vi "Actor Core.vi"(8 "error in":errorcluster, 11 "SinglePhotonInterferenceUI in":refnum<class "SinglePhotonInterferenceUI.lvclass">) -> (0 "error out":errorcluster, 3 "Actor out":refnum<class "Actor.lvclass">)   [LabVIEW 2023, in "SinglePhoton Library.lvlib" / "SinglePhotonInterferenceUI.lvlib" / "SinglePhotonInterferenceUI.lvclass"]
doc: "(<B>Filename</B>: Actor Framework.lvlib:Actor.lvclass:Actor Core.vi)\n\nReceives messages to the actor, reacts to them, and initiates any error handling that may shut the actor down.\n\nDescendant classes may override this VI to append parallel tasks for the actor to complete while it handles messages. Overrides use the Call Parent Class Method node."
uses:
  SinglePhotonInterferenceUI.lvclass
  C:/Program Files/National Instruments/LabVIEW 2023/vi.lib/ActorFramework/Actor/Actor.lvclass
  <vilib>/ActorFramework/Actor/Actor.lvclass
  ConcreteClasses/ConcreteInstrumentClasses/Multiharp/Multiharp/Types/MH_InputChannel.ctl
  ConcreteClasses/ConcreteInstrumentClasses/Multiharp/Multiharp/_lib/PQ/MultiHarp/MH_MeasMode.ctl
  <vilib>/ActorFramework/Message Enqueuer/Message Enqueuer.lvclass
  ConcreteClasses/ConcreteInstrumentClasses/Multiharp/Multiharp/Types/MH_UIThread_Data_SPI.ctl
  ConcreteClasses/ConcreteInstrumentClasses/Multiharp/Multiharp/_lib/PQ/MultiHarp/MH_InitInfo.ctl
  ConcreteClasses/ConcreteInstrumentClasses/Multiharp/Multiharp/Types/MH_SetInpChanData.ctl
  ConcreteClasses/ConcreteInstrumentClasses/Multiharp/Multiharp/Types/MH_SetInpChanCmds.ctl
  ConcreteClasses/ConcreteInstrumentClasses/Multiharp/Multiharp/Multiharp/Multiharp.lvclass
  <vilib>/ActorFramework/Actor/Actor.lvclass/Actor.ctl
  <vilib>/ActorFramework/Message Enqueuer/Message Enqueuer.lvclass/Message Enqueuer.ctl
  SinglePhotonInterferenceUI.lvclass/SinglePhotonInterferenceUI.ctl
  ConcreteClasses/ConcreteInstrumentClasses/Multiharp/Multiharp/Multiharp Messages/MH_Init Msg/MH_Init Msg.lvclass/MH_Init Msg.ctl
  ConcreteClasses/ConcreteInstrumentClasses/Multiharp/Multiharp/Multiharp Messages/SetInputChannels Msg/SetInputChannels Msg.lvclass/SetInputChannels Msg.ctl
  SPIController/SPIController Messages/MeasurementFinished Msg/MeasurementFinished Msg.lvclass/MeasurementFinished Msg.ctl
  ConcreteClasses/ConcreteInstrumentClasses/Multiharp/Multiharp/Multiharp Messages/SetSyncDivider Msg/SetSyncDivider Msg.lvclass/SetSyncDivider Msg.ctl
  ConcreteClasses/ConcreteInstrumentClasses/Multiharp/Multiharp/Multiharp Messages/SetSyncOffset Msg/SetSyncOffset Msg.lvclass/SetSyncOffset Msg.ctl
  ConcreteClasses/ConcreteInstrumentClasses/Multiharp/Multiharp/Multiharp Messages/SetSyncTrigger Msg/SetSyncTrigger Msg.lvclass/SetSyncTrigger Msg.ctl
  ConcreteClasses/ConcreteInstrumentClasses/Multiharp/Multiharp/Multiharp Messages/SetSyncDeadTime Msg/SetSyncDeadTime Msg.lvclass/SetSyncDeadTime Msg.ctl
  ConcreteClasses/ConcreteInstrumentClasses/Multiharp/Multiharp/Multiharp Messages/SetHistogramParameter Msg/SetHistogramParameter Msg.lvclass/SetHistogramParameter Msg.ctl
  ConcreteClasses/ConcreteInstrumentClasses/Multiharp/Multiharp/Multiharp Messages/MH_SetHistoOnOff Msg/MH_SetHistoOnOff Msg.lvclass/MH_SetHistoOnOff Msg.ctl
  <vilib>/ActorFramework/Message Enqueuer/Init from Existing Queue.vi
  <vilib>/ActorFramework/Message Enqueuer/Enqueue.vi
  ConcreteClasses/ConcreteInstrumentClasses/Multiharp/Multiharp/Multiharp Messages/MH_Init Msg/MH_Init Msg.lvclass
  C:/Program Files/National Instruments/LabVIEW 2023/vi.lib/ActorFramework/Message/Message.lvclass
  ConcreteClasses/ConcreteInstrumentClasses/Multiharp/Multiharp/Multiharp Messages/SetInputChannels Msg/SetInputChannels Msg.lvclass
  SPIController/SPIController Messages/MeasurementFinished Msg/MeasurementFinished Msg.lvclass
  ConcreteClasses/ConcreteInstrumentClasses/Multiharp/Multiharp/Multiharp Messages/StopMeasurement Msg/StopMeasurement Msg.lvclass
  ConcreteClasses/ConcreteInstrumentClasses/Multiharp/Multiharp/Multiharp Messages/SetSyncDivider Msg/SetSyncDivider Msg.lvclass
  ConcreteClasses/ConcreteInstrumentClasses/Multiharp/Multiharp/Multiharp Messages/SetSyncOffset Msg/SetSyncOffset Msg.lvclass
  ConcreteClasses/ConcreteInstrumentClasses/Multiharp/Multiharp/Multiharp Messages/SetSyncTrigger Msg/SetSyncTrigger Msg.lvclass
  ConcreteClasses/ConcreteInstrumentClasses/Multiharp/Multiharp/Multiharp Messages/SetSyncDeadTime Msg/SetSyncDeadTime Msg.lvclass
  ConcreteClasses/ConcreteInstrumentClasses/Multiharp/Multiharp/Multiharp Messages/SetHistogramParameter Msg/SetHistogramParameter Msg.lvclass
  ConcreteClasses/ConcreteInstrumentClasses/Multiharp/Multiharp/Multiharp Messages/MH_SetHistoOnOff Msg/MH_SetHistoOnOff Msg.lvclass
  <vilib>/ActorFramework/Stop Msg/Stop Msg.lvclass
  <vilib>/Utility/error.llb/Error Cluster From Error Code.vi
  ConcreteClasses/ConcreteInstrumentClasses/Multiharp/Multiharp/_lib/PQ/MultiHarp/mhlib_x86_x64_AnyThread.llb/MH_DllPath_global.vi
  <vilib>/ActorFramework/Message Priority Queue/Priority Enqueue.vi
  <vilib>/ErrorRing/Error Ring.xnode
  typedefs/typedefs.lvlib
panel:
  in  "MH_UIThread_Data":T1={"Init Info"={"Library Version"="", "Serial No."="", "Model"="", "Partnum"="", "Version"="", "features"=0, "nchannels"=0, "Base Resolution"=0.0, "Bin Steps"=0}, "DevIdx"=0, "SyncDivider"=1, "SyncOffset"=0, "SyncLevel"=50, "Channels"=[], "CurrentChannels"=[], "AcqTime"=1, "Binning"=1, "HistoOffset"=1, "HistoLen"=1024, "StopOvl."=FALSE, "OvlLevel"=1024, "SyncEdge"=10, "StartMeas"=FALSE, "HistoLength"=0, "Resolution"=0.0, "Run cont."=FALSE, "Status"="", "SyncRate"=0, "BitShift"=0, "HistoAcqTime"=0.0, "SyncRateStart"=0, "UseDeadTime"=FALSE, "SyncDeadTime"=800, "SetInpChan"=[], "max value"=[], "CoincidenceArray"=[], "Histo On"=FALSE, "Mode"=0, "Scanning"=FALSE, "Last Move"=FALSE, "Coincidence Window"=0.0, "Max Triggers"=0, "Coincidence Delays"=[], "T2 Coincidences Array"=[], "Clear Graph"=FALSE, "File Save Path"=path "", "T2 Coincidence Cluster"={"Coincidences"=[], "Mean"=[], "Sqrt(mean)"=[], "Stdev"=[]}, "Acquisitions"=0, "HR Array"=[], "Ext. Scanning"=FALSE, "AllanVariance"=[]} {"Acquisitions" min=0 max=100000000 step=1; "T2 Coincidence Cluster"."Stdev" format="%0.2f"; "T2 Coincidence Cluster"."Mean" format="%0.2f"; "Mode" items=["HIST"=0, "T2"=2, "T3"=3]; "SyncDeadTime" min=800 max=160000 step=1; "SyncEdge" items=["falling", "rising"]; "SyncDivider" items=["1", "2", "4", "8", "16"]; "SyncOffset" min=0 max=100000 step=1; "SyncLevel" min=0 max=800 step=1; "AcqTime" min=1 max=360000 step=1; "Binning" items=["1", "2", "4", "8", "16", "32", "64", "128", "256", "512", "1024", "2048", "4096", "8192", "16384", "32768", "65536", "131072", "262144", "524288", "1048576", "2097152", "4194304", "8388608", "16777216", "3355443225"]; "HistoOffset" min=0 max=500 step=1; "HistoLen" min=1024 max=65536 step=1024; "Channels"."DeadTime" min=800 max=160000 step=1; "Channels"."Edge" items=["falling", "rising"]; "Channels"."Offset" min=-100000 max=100000 step=10; "Channels"."Level" min=-1200 max=1200 step=1}
  out "Self Enqueuer":refnum<class "Message Enqueuer.lvclass">
  out "Caller Enqueuer":refnum<class "Message Enqueuer.lvclass">
  out "Multiharp Enqueuer":refnum<class "Message Enqueuer.lvclass">
  out "T2 Coincidence Cluster.Coincidences":i32[][](graph)
  out "AllanVariance":dbl[][](graph)
  out "syncrate":i32
  in  "Histograms On":bool
  in  "Acquisitions":u32=1 min=1 max=5000 step=1
  out "T2 Coincidence Cluster":T7 {"Stdev" format="%0.2f"; "Mean" format="%0.2f"}
  in  "FileName":string
  in  "Path":path
  in  "Clear Graph":bool
  in  "Coincidence Delays":dbl[](array[numeric])
  in  "Max Triggers":i32
  in  "Coincidence Window":dbl
  in  "Mode":T6=2 items=["HIST"=0, "T2"=2, "T3"=3]
  in  "HistoLength":i32(ring)=6 caption="Num Bins" items=["1024", "2048", "4096", "8192", "16384", "32768", "65536"]
  out "Status":string="Readout Rate: 8.6 Hz\t\tTotal Counts:\t\tCh. 1: 0 cnts.\t\tCh. 2: 1962112 cnts.\t\tCh. 3: 0 cnts.\t\tCh. 4: 1962112 cnts.\t\tCh. 5: 0 cnts.\t\tCh. 6: 1962112 cnts.\t\tCh. 7: 0 cnts.\t\tCh. 8: 1962112 cnts.\t\tCh. 9: 1962113 cnts.\t\tCh.10: 0 cnts.\t\tCh.11: 1962113 cnts.\t\tCh.12: 0 cnts.\t\tCh.13: 1962113 cnts.\t\tCh.14: 0 cnts.\t\tCh.15: 1962113 cnts.\t\tCh.16: 1962113 cnts.\t\t"
  out "CountRates":i32[](graph)
  out "SyncRate":string="Sync Rate: 4999950 cps\n"
  out "OverFlow":bool caption="Overflow:"
  out "HistoGraph":T8(graph)={0.0, "Resolution"=0.08, "Histograms"=[]}
  in  "AllChannels":T9={"Enable"=TRUE, "Offset"=0, "Level"=20, "Edge"=0, "DeadTime"=1000, "UseDeadTime"=FALSE, "SetEnableAllChan"=TRUE, "SetEdgeAllChan"=TRUE, "SetLevelAllChan"=TRUE, "SetOffsetAllChan"=TRUE, "SetUseDTAllChan"=TRUE, "SetDeadTAllChan"=TRUE} {"DeadTime" min=800 max=160000 step=1; "Edge" items=["falling", "rising"]; "Offset" min=-100000 max=100000 step=10; "Level" min=-1200 max=1200 step=1}
  in  "Scale":enum32{"Item 0", "Item 1"}(radio)
  in  "Run continuously":enum32{"Running Mode", "Item 1"}(radio) caption="Acquisition"
  in  "Start":bool
  in  "OvlLevel":u32=4294967295 caption="Ovl.Level" min=1 step=1
  in  "StopOvl.":bool=TRUE
  in  "AcqTime":i32=1000 caption="Acqu.           ms" min=1 max=3600000 step=1
  in  "HistoOffset":i32 caption="Offset            ns" min=0 max=100000000 step=1
  in  "Binning":i32(ring) caption="Resol.            ps" items=["10", "20", "40", "80", "160", "320", "640", "1280", "2560", "5120", "10240", "20480", "40960", "81920", "163840", "327680", "655360", "1310720", "2621440", "5242880", "10485760", "20971520", "41943040"]
  in  "UseDeadTime":bool caption="Use DT."
  in  "SyncDeadTime":i32=1000 caption="Dead T.   ps" min=800 max=160000 step=1
  in  "SyncLevel":i32=-100 caption="Level      mV" min=-1200 max=1200 step=1
  in  "SyncEdge":i32(ring) caption="Edge" items=["falling", "rising"]
  in  "SyncOffset":i32 caption="Offset      ps" min=-100000 max=100000 step=10
  in  "SyncDivider":i32(ring) caption="Divider" items=["1", "2", "4", "8", "16"]
  in  "Channels":T3[](array[typedef])=[{"Name"="Inp.Chan 1", "Enable"=TRUE, "Edge"=0, "Level"=-100, "Offset"=0, "UseDeadTime"=FALSE, "DeadTime"=1000}, {"Name"="Inp.Chan 2", "Enable"=TRUE, "Edge"=0, "Level"=-100, "Offset"=0, "UseDeadTime"=FALSE, "DeadTime"=1000}, {"Name"="Inp.Chan 3", "Enable"=TRUE, "Edge"=0, "Level"=-100, "Offset"=0, "UseDeadTime"=FALSE, "DeadTime"=1000}, {"Name"="Inp.Chan 4", "Enable"=TRUE, "Edge"=0, "Level"=-100, "Offset"=0, "UseDeadTime"=FALSE, "DeadTime"=1000}, {"Name"="Inp.Chan 5", "Enable"=TRUE, "Edge"=0, "Level"=-100, "Offset"=0, "UseDeadTime"=FALSE, "DeadTime"=1000}, {"Name"="Inp.Chan 6", "Enable"=TRUE, "Edge"=0, "Level"=-100, "Offset"=0, "UseDeadTime"=FALSE, "DeadTime"=1000}, {"Name"="Inp.Chan 7", "Enable"=TRUE, "Edge"=0, "Level"=-100, "Offset"=0, "UseDeadTime"=FALSE, "DeadTime"=1000}, {"Name"="Inp.Chan 8", "Enable"=TRUE, "Edge"=0, "Level"=-100, "Offset"=0, "UseDeadTime"=FALSE, "DeadTime"=1000}, {"Name"="Inp.Chan 9", "Enable"=TRUE, "Edge"=0, "Level"=-100, "Offset"=0, "UseDeadTime"=FALSE, "DeadTime"=1000}, {"Name"="Inp.Chan 10", "Enable"=TRUE, "Edge"=0, "Level"=-100, "Offset"=0, "UseDeadTime"=FALSE, "DeadTime"=1000}, {"Name"="Inp.Chan 11", "Enable"=TRUE, "Edge"=0, "Level"=-100, "Offset"=0, "UseDeadTime"=FALSE, "DeadTime"=1000}, {"Name"="Inp.Chan 12", "Enable"=TRUE, "Edge"=0, "Level"=-100, "Offset"=0, "UseDeadTime"=FALSE, "DeadTime"=1000}, {"Name"="Inp.Chan 13", "Enable"=TRUE, "Edge"=0, "Level"=-100, "Offset"=0, "UseDeadTime"=FALSE, "DeadTime"=1000}, {"Name"="Inp.Chan 14", "Enable"=TRUE, "Edge"=0, "Level"=-100, "Offset"=0, "UseDeadTime"=FALSE, "DeadTime"=1000}, {"Name"="Inp.Chan 15", "Enable"=TRUE, "Edge"=0, "Level"=-100, "Offset"=0, "UseDeadTime"=FALSE, "DeadTime"=1000}, {"Name"="Inp.Chan 16", "Enable"=TRUE, "Edge"=0, "Level"=-100, "Offset"=0, "UseDeadTime"=FALSE, "DeadTime"=1000}] {"DeadTime" min=800 max=160000 step=1; "Edge" items=["falling", "rising"]; "Offset" min=-100000 max=100000 step=10; "Level" min=-1200 max=1200 step=1}
  in  "Init Multiharp":bool
  in  "stop":bool
  out "VI":refnum<vi>
  out "Heralding Ratio":dbl[][](graph)
  out "Coincidence Array":dbl[][](graph)
  # "Sync"
  # "Histogram"
  # "All Channels"
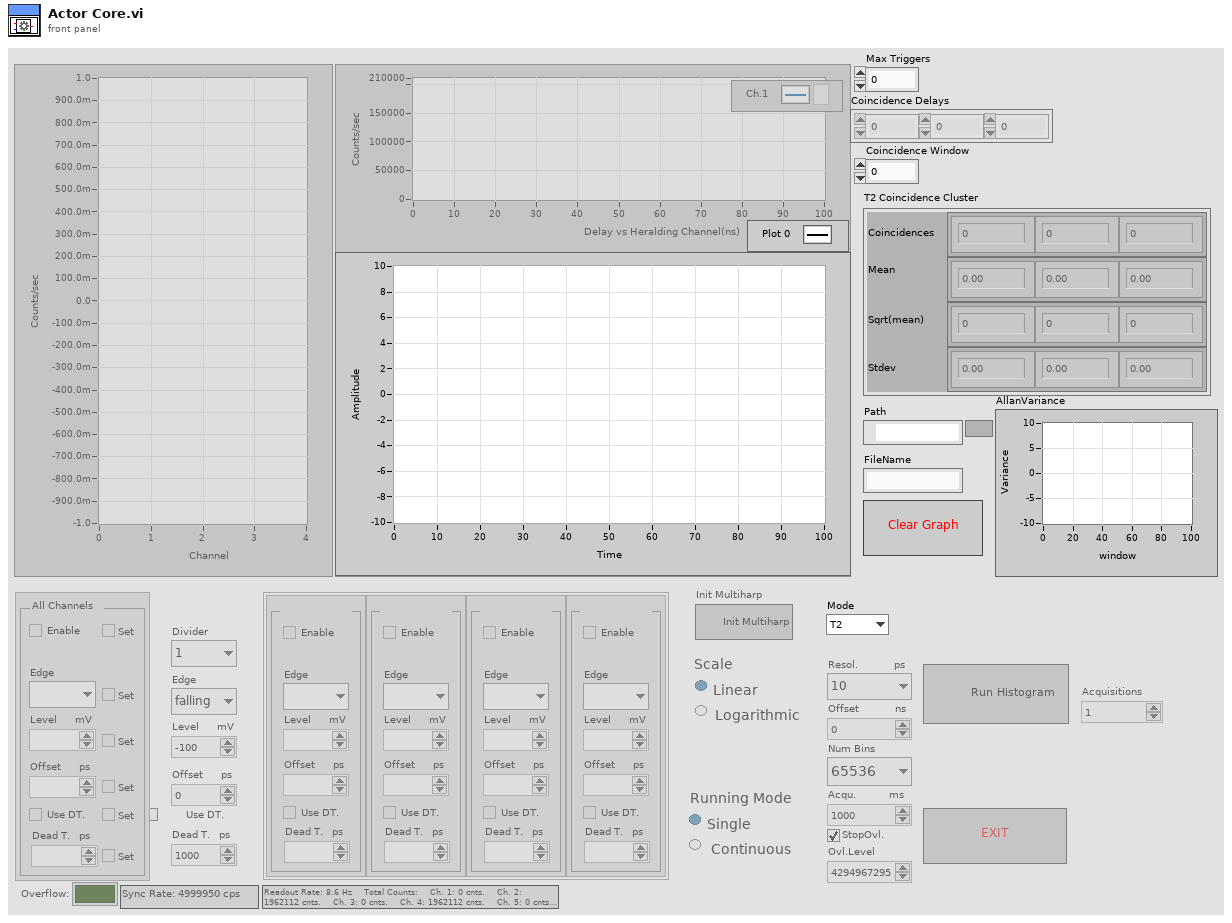
[diagram p1: front panel]
types:
  T1 = typedef "MH_UIThread_Data_SPI.ctl" = cluster{"Init Info":T2, "DevIdx":i32, "SyncDivider":i32, "SyncOffset":i32, "SyncLevel":i32, "Channels":T3[], "CurrentChannels":i32[], "AcqTime":i32, "Binning":i32, "HistoOffset":i32, "HistoLen":i32, "StopOvl.":bool, "OvlLevel":u32, "SyncEdge":i32, "StartMeas":bool, "HistoLength":i32, "Resolution":dbl, "Run cont.":bool, "Status":string, "SyncRate":i32, "BitShift":i32, "HistoAcqTime":dbl, "SyncRateStart":i32, "UseDeadTime":bool, "SyncDeadTime":i32, "SetInpChan":T4[], "max value":u32[], "CoincidenceArray":u32[][], "Histo On":bool, "Mode":T6, "Scanning":bool, "Last Move":bool, "Coincidence Window":dbl, "Max Triggers":i32, "Coincidence Delays":dbl[], "T2 Coincidences Array":i32[][], "Clear Graph":bool, "File Save Path":path, "T2 Coincidence Cluster":cluster{"Coincidences":u32[], "Mean":dbl[], "Sqrt(mean)":dbl[], "Stdev":dbl[]}, "Acquisitions":i32, "HR Array":sgl[][], "Ext. Scanning":bool, "AllanVariance":dbl[][]}
  T2 = typedef "typedefs.lvlib/MH_InitInfo.ctl" = cluster{"Library Version":string, "Serial No.":string, "Model":string, "Partnum":string, "Version":string, "features":i32, "nchannels":i32, "Base Resolution":dbl, "Bin Steps":i32}
  T3 = typedef "MH_InputChannel.ctl" = cluster{"Name":string, "Enable":bool, "Edge":i32, "Level":i32, "Offset":i32, "UseDeadTime":bool, "DeadTime":i32}
  T4 = typedef "MH_SetInpChanData.ctl" = cluster{"Channel":i32, "Cmds":T5[], "Changed":cluster{"Name":bool, "Enable":bool, "Edge":bool, "Level":bool, "Offset":bool, "UseDeadTime":bool, "DeadTime":bool}}
  T5 = typedef "MH_SetInpChanCmds.ctl" = enum16{"SetInpChanEnable", "SetInpChanOffset", "SetInpChanDeadTime", "SetInpChanTrg"}
  T6 = typedef "MH_MeasMode.ctl" = i32
  T7 = cluster{"Coincidences":dbl[], "Mean":dbl[], "Sqrt(mean)":dbl[], "Stdev":dbl[]}
  T8 = cluster{dbl, "Resolution":dbl, "Histograms":u32[][]}
  T9 = cluster{"Enable":bool, "Offset":i32, "Level":i32, "Edge":i32, "DeadTime":i32, "UseDeadTime":bool, "SetEnableAllChan":bool, "SetEdgeAllChan":bool, "SetLevelAllChan":bool, "SetOffsetAllChan":bool, "SetUseDTAllChan":bool, "SetDeadTAllChan":bool}
  T10 = enum8{"Enabled", "Disabled", "Disabled and Grayed Out"}
  T11 = typedef "MH_InputChannel2.ctl" = cluster{"Name":string, "Enable":bool, "Edge":i32, "Level":i32, "Offset":i32, "UseDeadTime":bool, "DeadTime":i32}
  T12 = cluster{"Coincidences":u32[], "Mean":dbl[], "Sqrt(mean)":dbl[], "Stdev":dbl[]}
  T13 = cluster{"[0]":bool, "[1]":bool, "[2]":bool, "[3]":bool, "[4]":bool, "[5]":bool}
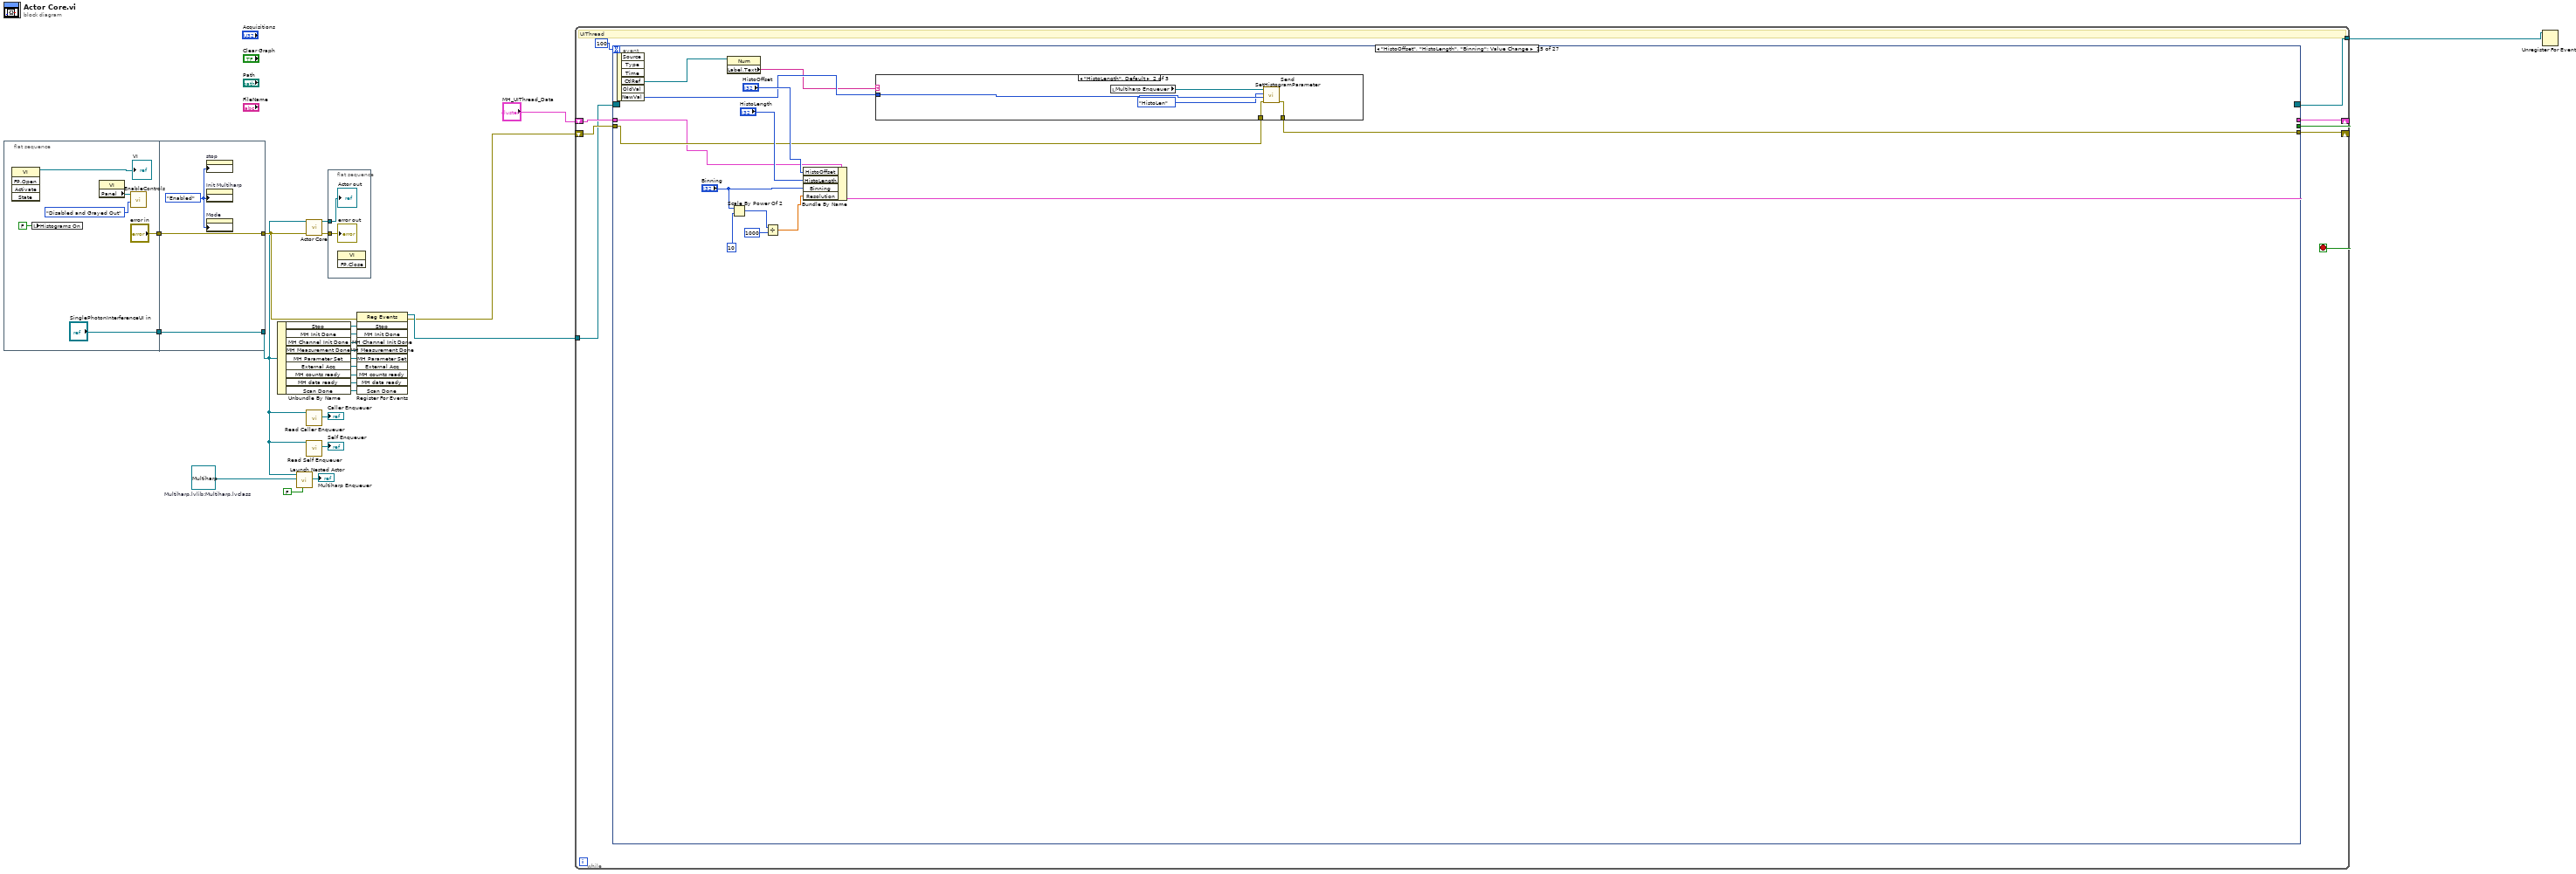
[diagram p0: block diagram]
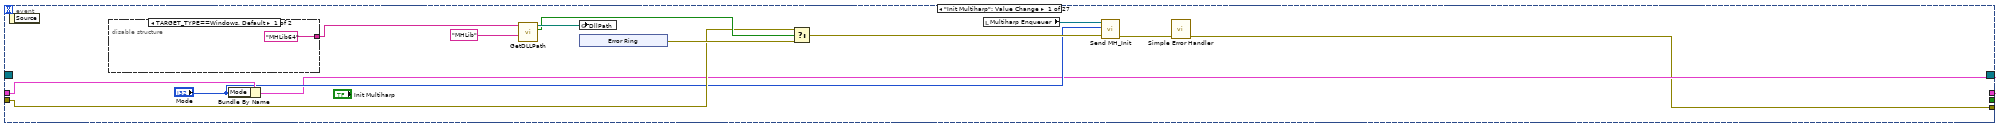
[diagram p2: hidden frame]
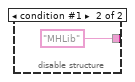
[diagram p3: hidden frame]
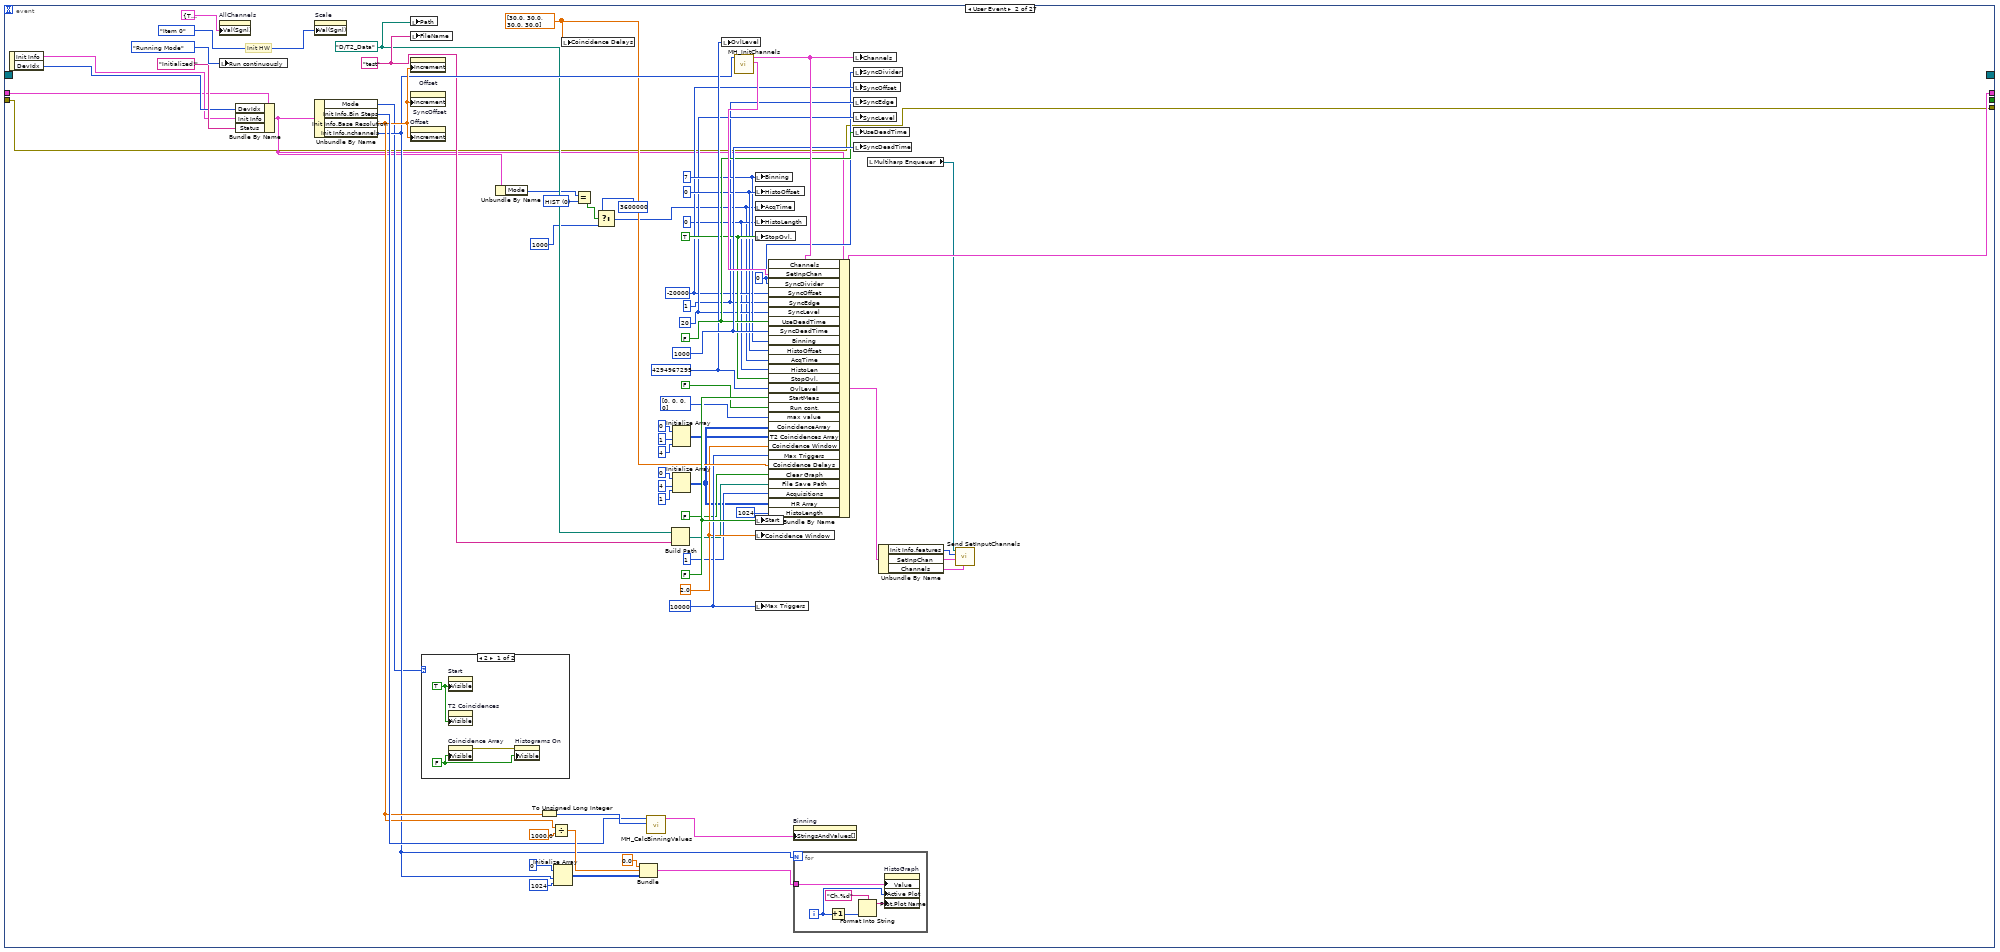
[diagram p4: hidden frame]
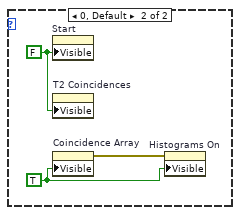
[diagram p5: hidden frame]
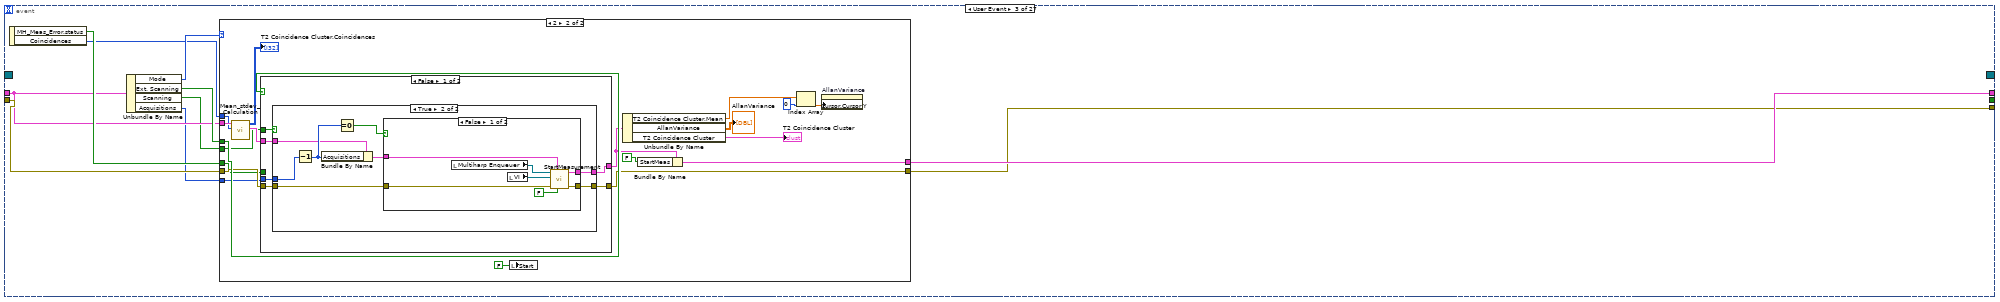
[diagram p6: hidden frame]
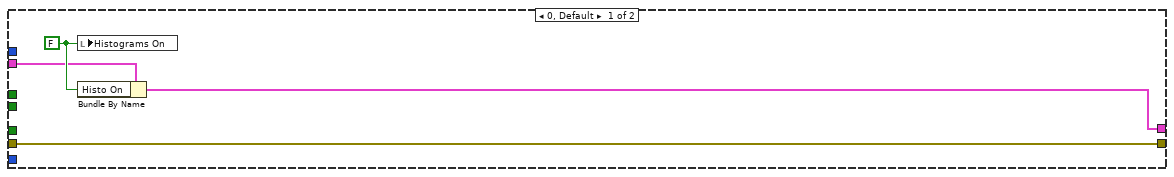
[diagram p7: hidden frame]
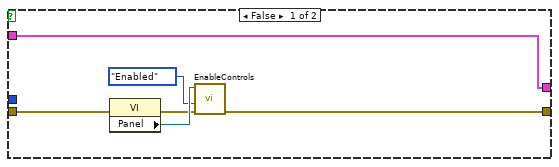
[diagram p8: hidden frame]
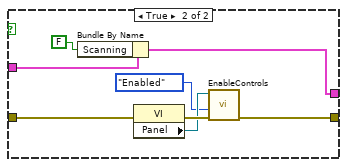
[diagram p9: hidden frame]
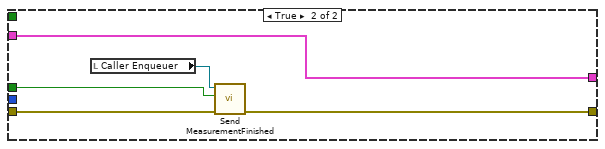
[diagram p10: hidden frame]
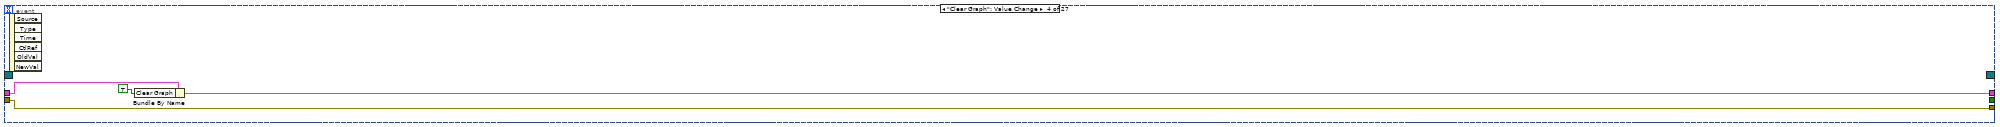
[diagram p11: hidden frame]
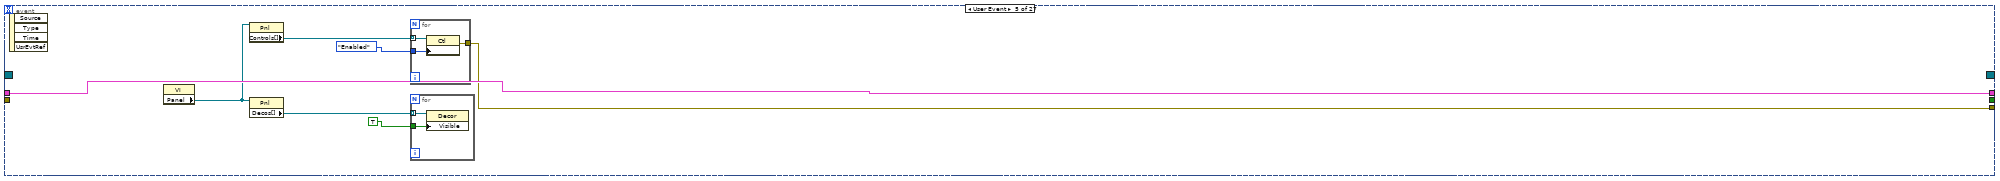
[diagram p12: hidden frame]
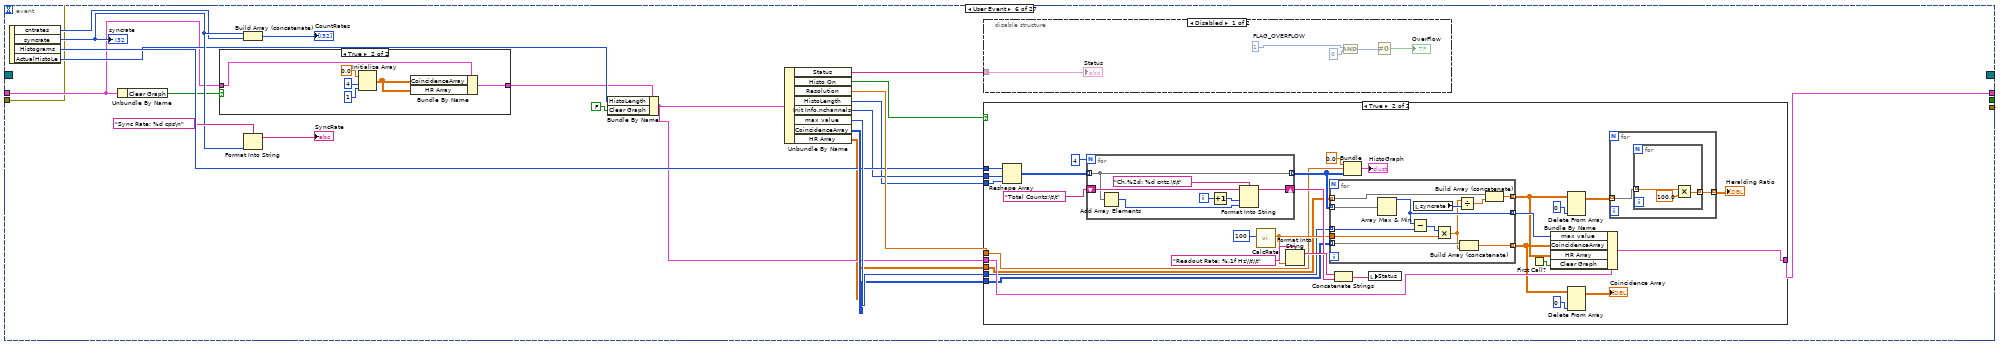
[diagram p13: hidden frame]
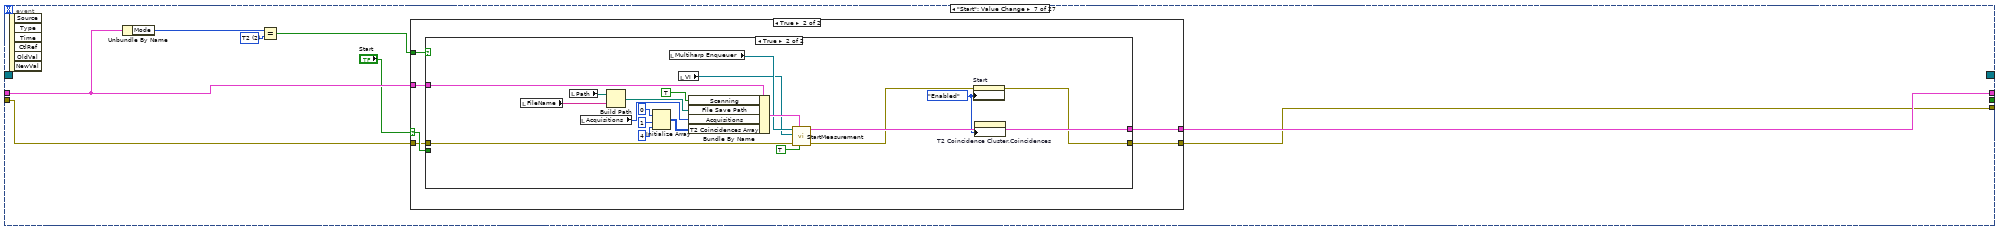
[diagram p17: hidden frame]
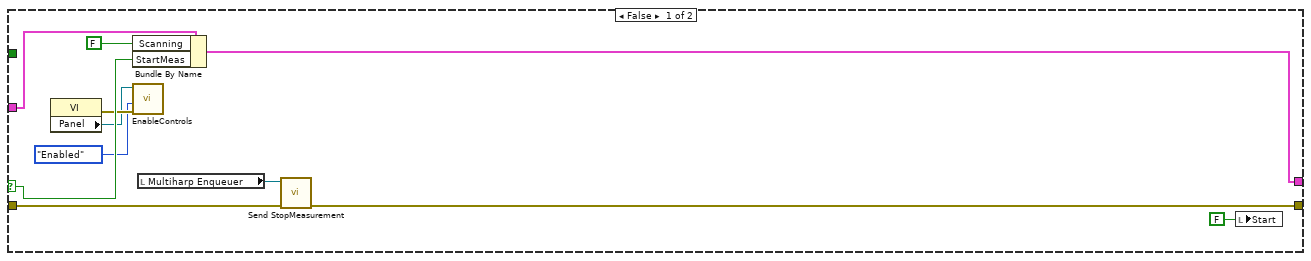
[diagram p18: hidden frame]
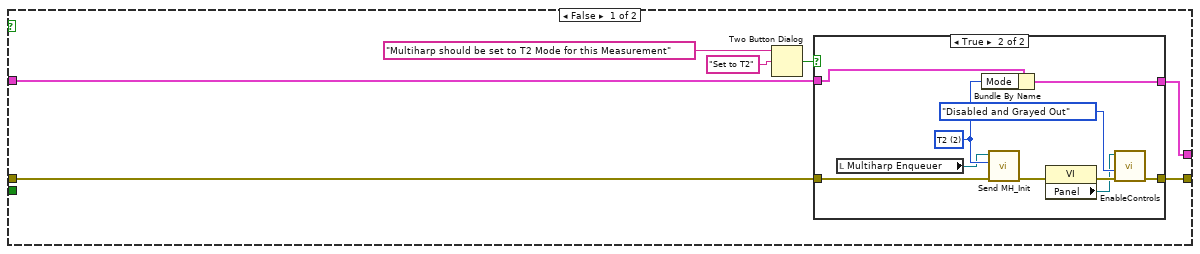
[diagram p19: hidden frame]
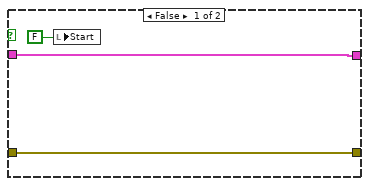
[diagram p20: hidden frame]
diagram:
  w9 = refnum<class "Multiharp.lvclass"> refnum  # Multiharp.lvlib:Multiharp.lvclass
  n1 = flat-sequence {
    tunnel: ["error in"] -> w8
    tunnel: ["SinglePhotonInterferenceUI in"] -> w7
    tunnel: [w32] -> w3
    tunnel: [w33] -> w11
    tunnel: w8 -> [w33]
    tunnel: w7 -> [w32]
    frame #0 {
      n2 = invoke class="VI" method="FP.Open"() -> (reference out=→"VI":refnum<vi>)  [unwired: 5 in, 4 out]
      n3 = local write "Histograms On"(FALSE ("Histograms On")) -> ()
      n4 = property class="VI"() -> ("Panel"=w27:refnum<vi>)  [unwired: 2 in, 2 out]
      n5 = call "EnableControls.vi"("Disabled"=T10."Disabled and Grayed Out", "Panel in"=w27) -> ()  [unwired: 9 in, 1 out]
    }
    frame #1 {
      w31 = T10."Enabled" ("Disabled")
      n6 = property on="stop" class="Bool"("DisabledEnum"=w31) -> ()  [unwired: 2 in, 2 out]
      n7 = property on="Init Multiharp" class="Bool"("DisabledEnum"=w31) -> ()  [unwired: 2 in, 2 out]
      n8 = property on="Mode" class="Ring (strict)"("DisabledEnum"=w31) -> ()  [unwired: 2 in, 2 out]
    }
  }
  n9 = Unbundle By Name(w3) -> ("Stop"=w21:refnum<user-event>, "MH Init Done"=w20:refnum<user-event>, "MH Channel Init Done"=w19:refnum<user-event>, "MH Measurement Done"=w18:refnum<user-event>, "MH Parameter Set"=w17:refnum<user-event>, "External Acq"=w16:refnum<user-event>, "MH counts ready"=w14:refnum<user-event>, "MH data ready"=w13:refnum<user-event>, "Scan Done"=w1:refnum<user-event>)
  n10 = call <vilib>:"Launch Nested Actor.vi"("Open Actor Core front panel? (F)"=FALSE, "Nested Actor"=w9, "Caller Actor in"=w3) -> ("Nested Actor's Enqueuer"=→"Multiharp Enqueuer":refnum<class "Message Enqueuer.lvclass">)  [unwired: 6 in, 2 out]
  n11 = call-parent "Actor Core.vi"("error in"=w11, "Actor in"=w3) -> ("error out"=w24:errorcluster, "Actor out"=w23:refnum<class "Actor.lvclass">)  [unwired: 8 in]
  n12 = call <vilib>:"Read Caller Enqueuer.vi"("Actor"=w3) -> ("Caller Enqueuer"=→"Caller Enqueuer":refnum<class "Message Enqueuer.lvclass">)  [unwired: 10 in]
  n13 = call <vilib>:"Read Self Enqueuer.vi"("Actor"=w3) -> ("Self Enqueuer"=→"Self Enqueuer":refnum<class "Message Enqueuer.lvclass">)  [unwired: 10 in]
  n14 = flat-sequence {
    tunnel: w24 -> [w35]
    tunnel: w23 -> [w34]
    frame #0 {
      n15 = invoke class="VI" method="FP.Close"() -> ()  [unwired: 3 in, 3 out]
      "error out" <- w35
      "Actor out" <- w34
    }
  }
  n16 = register-events(error in=w11, w21, w20, w19, w18, w17, w16, w14, w13, w1) -> (reference out=w22:refnum<event-registration>, error out=w10:errorcluster)  [unwired: 1 in]
  n17 = while {
    shift-right: [w43] -> _
    shift-left: "MH_UIThread_Data" -> [w42]
    shift-right: [w39] -> _
    shift-left: w10 -> [w41]
    tunnel: w22 -> [w40]
    tunnel: [w38] -> w15
    stop <- w36 stop-if-true
    # "UIThread"
    n18 = event shown="[14] \"HistoOffset\", \"HistoLength\", \"Binning\": Value Change" {
      selector: w40 -> [_ _ _ _ _ _ _ _ _ _ _ _ _ _ _ _ _ _ _ _ _ _ _ _ _ _ _]
      dyn-events: [_ _ _ _ _ _ _ _ _ _ _ _ _ _ _ _ _ _ _ _ _ _ _ _ _ _ _] -> w38
      timeout: 100 -> [_ _ _ _ _ _ _ _ _ _ _ _ _ _ _ _ _ _ _ _ _ _ _ _ _ _ _]
      tunnel: [w46 w93 w149 w214 w224 w248 w326 w391 w443 w458 w512 w520 w529 w542 w561 w583 w625 w632 w635 w644 w650 w653 w657 w663 w665 w667 w672] -> w43
      tunnel: w42 -> [w48 w97 w145 w217 w224 w234 w325 w390 w446 w451 w509 w516 w526 w534 w553 w587 w626 w628 w636 w639 w651 w653 w657 w663 w665 w667 w672]
      tunnel: [w44 w72 w143 w215 w218 w230 w319 w385 w433 w450 w508 w517 w524 w530 w554 w578 w623 w627 w633 w640 w645 w652 w658 w661 w664 w666 w668] -> w39
      tunnel: w41 -> [w49 w72 w147 w215 _ w230 w320 w386 w445 w450 _ w517 w524 w531 w555 w584 w623 w627 w633 w640 w645 w652 w658 w661 w664 w666 w668]
      tunnel: [_ _ _ _ _ _ _ _ _ _ _ _ _ _ _ _ _ _ _ _ _ _ _ TRUE _ _ _] -> w36
      event "Init Multiharp": Value Change {
        n19 = event-data() -> ()  [unwired: 1 in, 1 out]
        n20 = disable-structure shown="TARGET_TYPE==Windows, Default" {
          disable-tunnel: ["MHLib64" ("name or relative path") "MHLib" ("name or relative path")] -> w52
          frame condition #0 (active) {
          }
          frame condition #1 {
          }
        }
        n21 = Bundle By Name(cluster=w48, "Mode"="Mode") -> (w46:T1)
        n22 = call "GetDLLPath.vi"("DllName_32bit"="MHLib" ("name or relative path"), "DllName_64bit"=w52) -> ("file exists?"=w54:bool, "DLLPath"=w55:path)  [unwired: 8 in]
        n23 = global write "MH_DllPath_global.vi" "DllPath"(w55) -> ()
        n24 = xnode "Error Ring"() -> ("error out"=w53:errorcluster)
        n25 = Select(t=w49, s=w54, f=w53) -> (s? t:f=w51:errorcluster)
        n26 = local read "Multiharp Enqueuer"() -> (w45:refnum<class "Message Enqueuer.lvclass">)
        n27 = call "Send MH_Init.vi"("error in (no error)"=w51, "Mode"="Mode", "Message Enqueuer"=w45) -> ("error out"=w50:errorcluster)  [unwired: 7 in, 1 out]
        n28 = call <vilib>:"Simple Error Handler.vi"("error in (no error)"=w50) -> ("error out"=w44:errorcluster)  [unwired: 4 in, 4 out]
      }
      event User Event {
        w69 = T6 0 items=["HIST"=0, "T2"=2, "T3"=3] ("y")
        w86 = "test" ("name or relative path")
        w85 = path "D:/T2_Data" ("base path")
        w89 = 2.0 ("Max Delay")
        w90 = 10000 ("Max Triggers")
        w91 = dbl[] [30.0, 30.0, 30.0, 30.0] ("Expected Delay")
        w121 = 1000 ("SyncDeadTime")
        w120 = FALSE ("UseDeadTime")
        w113 = FALSE ("StartMeas")
        w112 = u32 4294967295 ("OvlLevel")
        w111 = TRUE ("StopOvl.")
        w92 = 0 ("HistoLen")
        w110 = 0 ("HistoOffset")
        w109 = 7 ("Binning")
        w108 = 20 ("SyncLevel")
        w107 = 1 ("SyncZeroX")
        w106 = -20000 ("SyncOffset")
        w105 = 0 ("SyncDivider")
        # "Init HW"
        n29 = event-data() -> ("Init Info"=w99:T2, "DevIdx"=w100:i32)  [unwired: 1 in]
        n30 = property on="AllChannels" class="Clust (strict)"("Val(Sgnl)"=T9 {"Enable"=TRUE, "Offset"=0, "Level"=20, "Edge"=1, "DeadTime"=1000, "UseDeadTime"=FALSE, "SetEnableAllChan"=TRUE, "SetEdgeAllChan"=TRUE, "SetLevelAllChan"=TRUE, "SetOffsetAllChan"=TRUE, "SetUseDTAllChan"=TRUE, "SetDeadTAllChan"=TRUE} ("AllChannels")) -> ()  [unwired: 2 in, 2 out]
        n31 = local write "Run continuously"(enum32{"Running Mode", "Item 1"}."Running Mode" ("Run continuously")) -> ()
        n32 = Bundle By Name(cluster=w97, "DevIdx"=w100, "Init Info"=w99, "Status"="Initialized!") -> (w71:T1)
        n33 = property on="Scale" class="RadioBtnsControl (strict)"("Val(Sgnl)"=enum32{"Item 0", "Item 1"}."Item 0" ("Value (Signaling)")) -> ()  [unwired: 2 in, 2 out]
        n34 = Unbundle By Name(w71) -> ("Mode"=w83:T6, "Init Info.Bin Steps"=w102:i32, "Init Info.Base Resolution"=w101:dbl, "Init Info.nchannels"=w98:i32)
        n35 = local write "Path"(w85) -> ()
        n36 = local write "FileName"(w86) -> ()
        n37 = property on="Offset" class="DigNum (strict)"("Increment"=w101) -> ()  [unwired: 2 in, 2 out]
        n38 = property on="SyncOffset" class="DigNum (strict)"("Increment"=w101) -> ()  [unwired: 2 in, 2 out]
        n39 = property on="Offset" class="DigNum (strict)"("Increment"=w101) -> ()  [unwired: 2 in, 2 out]
        n40 = case shown="2" w83 {
          frame 2 {
            w132 = FALSE ("Visible")
            w130 = TRUE ("Visible")
            n41 = property on="Start" class="Bool (strict)"("Visible"=w130) -> ()  [unwired: 2 in, 2 out]
            n42 = property on="T2 Coincidences" class="WFGraph (strict)"("Visible"=w130) -> ()  [unwired: 2 in, 2 out]
            n43 = property on="Coincidence Array" class="WFGraph (strict)"("Visible"=w132) -> (error out=w131:errorcluster)  [unwired: 2 in, 1 out]
            n44 = property on="Histograms On" class="Bool (strict)"(error in=w131, "Visible"=w132) -> ()  [unwired: 1 in, 2 out]
          }
          frame 0, Default {
            w135 = TRUE ("Visible")
            w133 = FALSE ("Visible")
            n45 = property on="Start" class="Bool (strict)"("Visible"=w133) -> ()  [unwired: 2 in, 2 out]
            n46 = property on="T2 Coincidences" class="WFGraph (strict)"("Visible"=w133) -> ()  [unwired: 2 in, 2 out]
            n47 = property on="Coincidence Array" class="WFGraph (strict)"("Visible"=w135) -> (error out=w134:errorcluster)  [unwired: 2 in, 1 out]
            n48 = property on="Histograms On" class="Bool (strict)"(error in=w134, "Visible"=w135) -> ()  [unwired: 1 in, 2 out]
          }
        }
        n49 = Unbundle By Name(w71) -> ("Mode"=w70:T6)
        n50 = To Unsigned Long Integer(number=w101) -> (unsigned 32bit integer=w123:u32)
        n51 = Divide(x=w101, y=1000.0) -> (x/y=w128:dbl)
        n52 = Initialize Array(u32 0, w98, 1024 ("dimension size")) -> (w127:u32[][])
        n53 = local write "Coincidence Delays"(w91) -> ()
        n54 = Equal?(x=w70, y=w69) -> (x = y?=w68:bool)
        n55 = Select(t=3600000 ("AcqTime"), s=w68, f=1000 ("AcqTime")) -> (s? t:f=w67:i32)
        n56 = Bundle(0.0, w128, w127) -> (w126:cluster{dbl, dbl, u32[][]})  [unwired: 1 in]
        n57 = call "MH_CalcBinningValues.vi"("BaseResolution"=w123, "Bin Steps"=w102) -> ("BinningValues"=w129:cluster{"String":string, "Value":i32}[])  [unwired: 9 in]
        n58 = Build Path(base path=w85, name or relative path=w86) -> (appended path=w87:path)
        n59 = Initialize Array(0 ("dimension size"), 1 ("dimension size"), 4 ("dimension size")) -> (w74:i32[][])
        n60 = Initialize Array(0 ("dimension size"), 4 ("dimension size"), 1 ("dimension size")) -> (w80:i32[][])
        n61 = local write "OvlLevel"(w112) -> ()
        n62 = call "MH_InitChannels.vi"("nchannels"=w98) -> ("SetInpChan"=w124:T4[], "Channels"=w125:T11[])  [unwired: 9 in]
        n63 = local write "Binning"(w109) -> ()
        n64 = local write "HistoOffset"(w110) -> ()
        n65 = local write "AcqTime"(w67) -> ()
        n66 = local write "HistoLength"(w92) -> ()
        n67 = local write "StopOvl."(w111) -> ()
        n68 = local write "Start"(w113) -> ()
        n69 = local write "Coincidence Window"(w89) -> ()
        n70 = local write "Max Triggers"(w90) -> ()
        n71 = Bundle By Name(cluster=w71, "Channels"=w125, "SetInpChan"=w124, "SyncDivider"=w105, "SyncOffset"=w106, "SyncEdge"=w107, "SyncLevel"=w108, "UseDeadTime"=w120, "SyncDeadTime"=w121, "Binning"=w109, "HistoOffset"=w110, "AcqTime"=w67, "HistoLen"=w92, "StopOvl."=w111, "OvlLevel"=w112, "StartMeas"=w113, "Run cont."=FALSE, "max value"=u32[] [0, 0, 0, 0], "CoincidenceArray"=w80, "T2 Coincidences Array"=w74, "Coincidence Window"=w89, "Max Triggers"=w90, "Coincidence Delays"=w91, "Clear Graph"=FALSE, "File Save Path"=w87, "Acquisitions"=1, "HR Array"=w80, "HistoLength"=1024) -> (w93:T1)
        n72 = property on="Binning" class="Ring (strict)"("StringsAndValues[]"=w129) -> ()  [unwired: 2 in, 2 out]
        n73 = for {
          N: w98 -> [_]
          tunnel: w126 -> [w138]
          i -> [w137]
          n74 = Increment(x=w137) -> (x+1=w139:i32)
          n75 = Format Into String(format string="Ch.%d", w139) -> (resulting string=w136:string)  [unwired: 2 in, 1 out]
          n76 = property on="HistoGraph" class="WFGraph (strict)"("Value"=w138, "Active Plot"=w137, "Plot.Plot Name"=w136) -> ()  [unwired: 2 in, 2 out]
        }
        n77 = local write "Channels"(w125) -> ()
        n78 = local write "SyncDivider"(w105) -> ()
        n79 = local write "SyncOffset"(w106) -> ()
        n80 = local write "SyncEdge"(w107) -> ()
        n81 = local write "SyncLevel"(w108) -> ()
        n82 = local write "UseDeadTime"(w120) -> ()
        n83 = local write "SyncDeadTime"(w121) -> ()
        n84 = local read "Multiharp Enqueuer"() -> (w73:refnum<class "Message Enqueuer.lvclass">)
        n85 = Unbundle By Name(w93) -> ("Init Info.features"=w95:i32, "SetInpChan"=w96:T4[], "Channels"=w94:T3[])
        n86 = call "Send SetInputChannels.vi"("Channels"=w94, "SetInpChan"=w96, "features"=w95, "Message Enqueuer"=w73) -> ()  [unwired: 6 in, 2 out]
      }
      event User Event {
        n87 = event-data() -> ("MH_Meas_Error.status"=w146:bool, "Coincidences"=w144:i32[])  [unwired: 1 in]
        n88 = Unbundle By Name(w145) -> ("Mode"=w150:T6, "Ext. Scanning"=w148:bool, "Scanning"=w142:bool, "Acquisitions"=w141:i32)
        n89 = case shown="2" w150 {
          tunnel: [w154 w173] -> w149
          tunnel: w148 -> [_ w171]
          tunnel: w147 -> [w151 w170]
          tunnel: w146 -> [_ w169]
          tunnel: w145 -> [w152 w162]
          tunnel: w144 -> [_ w161]
          tunnel: w141 -> [_ w167]
          tunnel: [w151 w166] -> w143
          tunnel: w142 -> [_ w160]
          frame 0, Default {
            w153 = FALSE ("Histo On")
            n90 = local write "Histograms On"(w153) -> ()
            n91 = Bundle By Name(cluster=w152, "Histo On"=w153) -> (w154:T1)
          }
          frame 2 {
            n92 = call "Mean_stdev_Calculation.vi"("Coincidences"=w161, "MH_UIThread_Data in"=w162) -> ("MH_UIThread_Data out"=w163:T1, "T2 Coincidences"=→"T2 Coincidence Cluster.Coincidences":i32[][])  [unwired: 8 in]
            n93 = case shown="False" w171 {
              tunnel: w170 -> [w179 w213]
              tunnel: [w176 w210] -> w164
              tunnel: w169 -> [_ w212]
              tunnel: w167 -> [w177 _]
              tunnel: [w178 w211] -> w166
              tunnel: w163 -> [w175 w210]
              tunnel: w160 -> [w174 _]
              frame False {
                n94 = case shown="True" w174 {
                  tunnel: w179 -> [w181 w193]
                  tunnel: [w180 w192] -> w178
                  tunnel: w177 -> [_ w191]
                  tunnel: [w185 w189] -> w176
                  tunnel: w175 -> [w185 w186]
                  frame False {
                    n95 = property class="VI"(error in=w181) -> (error out=w183:errorcluster, "Panel"=w184:refnum<vi>)  [unwired: 1 in, 1 out]
                    n96 = call "EnableControls.vi"("error in (no error)"=w183, "Disabled"=T10."Enabled", "Panel in"=w184) -> ("error out"=w180:errorcluster)  [unwired: 8 in]
                  }
                  frame True {
                    n97 = Decrement(x=w191) -> (x-1=w188:i32)
                    n98 = Bundle By Name(cluster=w186, "Acquisitions"=w188) -> (w187:T1)
                    n99 = Equal To 0?(x=w188) -> (x = 0?=w190:bool)
                    n100 = case shown="False" w190 {
                      tunnel: w193 -> [w200 w205]
                      tunnel: [w199 w204] -> w192
                      tunnel: w187 -> [w197 w203]
                      tunnel: [w196 w202] -> w189
                      frame False {
                        n101 = local read "Multiharp Enqueuer"() -> (w194:refnum<class "Message Enqueuer.lvclass">)
                        n102 = local read "VI"() -> (w195:refnum<vi>)
                        n103 = call "StartMeasurement.vi"("First Measurement?"=FALSE, "MH_UIThread_Data"=w197, "error in (no error)"=w200, "VI reference"=w195, "Multiharp Enqueuer"=w194) -> ("error out"=w199:errorcluster, "MH_UIThread_Data"=w196:T1)  [unwired: 5 in]
                      }
                      frame True {
                        n104 = Bundle By Name(cluster=w203, "Scanning"=FALSE) -> (w202:T1)
                        n105 = property class="VI"(error in=w205) -> (error out=w208:errorcluster, "Panel"=w207:refnum<vi>)  [unwired: 1 in, 1 out]
                        n106 = call "EnableControls.vi"("error in (no error)"=w208, "Disabled"=T10."Enabled", "Panel in"=w207) -> ("error out"=w204:errorcluster)  [unwired: 8 in]
                      }
                    }
                  }
                }
              }
              frame True {
                n107 = local read "Caller Enqueuer"() -> (w209:refnum<class "Message Enqueuer.lvclass">)
                n108 = call "Send MeasurementFinished.vi"("error in (no error)"=w213, "Error"=w212, "Message Enqueuer"=w209) -> ("error out"=w211:errorcluster)  [unwired: 7 in, 1 out]
              }
            }
            n109 = local write "Start"(FALSE ("Start")) -> ()
            n110 = Unbundle By Name(w164) -> ("T2 Coincidence Cluster.Mean"=w158:dbl[], "AllanVariance"=→"AllanVariance":dbl[][], "T2 Coincidence Cluster"=→"T2 Coincidence Cluster":T12)
            n111 = Bundle By Name(cluster=w164, "StartMeas"=FALSE ("Histo On")) -> (w173:T1)
            n112 = Index Array(array=w158, index=0) -> (element=w157:dbl)
            n113 = property on="AllanVariance" class="WFGraph (strict)"("Cursor.Cursor Y"=w157) -> ()  [unwired: 2 in, 2 out]
          }
        }
      }
      event "Clear Graph": Value Change {
        n114 = event-data() -> ()  [unwired: 1 in, 6 out]
        n115 = Bundle By Name(cluster=w217, "Clear Graph"=TRUE) -> (w214:T1)
      }
      event User Event {
        n116 = event-data() -> ()  [unwired: 1 in, 4 out]
        n117 = property class="VI"() -> ("Panel"=w222:refnum<vi>)  [unwired: 2 in, 2 out]
        n118 = property class="Pnl"(reference=w222) -> ("Controls[]"=w221:refnum<vi>[])  [unwired: 1 in, 2 out]
        n119 = property class="Pnl"(reference=w222) -> ("Decos[]"=w223:refnum<vi>[])  [unwired: 1 in, 2 out]
        n120 = for {
          tunnel: w221 -> [w229] mode=indexing
          tunnel: T10."Enabled" ("Disabled") -> [w228]
          tunnel: [w227] -> w218
          n121 = property class="Ctl"(reference=w229, "DisabledEnum"=w228) -> (error out=w227:errorcluster)  [unwired: 1 in, 1 out]
        }
        n122 = for {
          tunnel: w223 -> [w226] mode=indexing
          tunnel: TRUE -> [w225]
          n123 = property class="Decor"(reference=w226, "Visible"=w225) -> ()  [unwired: 1 in, 2 out]
        }
      }
      event User Event {
        n124 = event-data() -> ("cntrates"=w243:i32[], "syncrate"=w244:i32, "Histograms"=w246:u32[], "ActualHistoLe"=w239:i32)  [unwired: 1 in]
        "syncrate" <- w244
        n125 = Unbundle By Name(w234) -> ("Clear Graph"=w235:bool)
        n126 = case shown="True" w235 {
          tunnel: w234 -> [w252 w257]
          tunnel: [w252 w258] -> w233
          frame False {
          }
          frame True {
            n127 = Initialize Array(0.0 ("element"), 4 ("dimension size"), 1 ("dimension size")) -> (w256:dbl[][])
            n128 = Bundle By Name(cluster=w257, "CoincidenceArray"=w256, "HR Array"=w256) -> (w258:T1)
          }
        }
        n129 = Build Array (concatenate)(w244, w243) -> (→"CountRates":i32[])
        n130 = Format Into String(format string="Sync Rate: %d cps\n", w244) -> (resulting string=→"SyncRate":string)  [unwired: 2 in, 1 out]
        n131 = Bundle By Name(cluster=w233, "HistoLength"=w239, "Clear Graph"=FALSE) -> (w237:T1)
        n132 = Unbundle By Name(w237) -> ("Status"=w236:string, "Histo On"=w247:bool, "Resolution"=w251:dbl, "HistoLength"=w238:i32, "Init Info.nchannels"=w240:i32, "max value"=w250:u32[], "CoincidenceArray"=w249:u32[][], "HR Array"=w231:sgl[][])
        n133 = disable-structure shown="Disabled" {
          disable-tunnel: w236 -> [w314 _]
          frame Disabled {
            w317 = 1  # FLAG_OVERFLOW
            n134 = And(x=w317, y=0) -> (x .and. y?=w318:i32)
            n135 = Not Equal To 0?(x=w318) -> (x != 0?=→"OverFlow":bool)
            "Status" <- w314
          }
          frame Enabled {
          }
        }
        n136 = case shown="True" w247 {
          tunnel: w246 -> [_ w277]
          tunnel: w251 -> [_ w276]
          tunnel: w250 -> [_ w271]
          tunnel: w249 -> [_ w269]
          tunnel: [w259 w275] -> w248
          tunnel: w237 -> [w259 w274]
          tunnel: w240 -> [_ w273]
          tunnel: w238 -> [_ w272]
          tunnel: w231 -> [_ w268]
          frame False {
          }
          frame True {
            n137 = Reshape Array(w277, w273, w272) -> (w283:u32[][])
            n138 = for {
              N: 4 -> [_]
              tunnel: [w307] -> w280 mode=indexing
              shift-right: [w309] -> w284
              shift-left: "Total Counts:\t\t" -> [w308]
              tunnel: w283 -> [w307] mode=indexing
              i -> [w313]
              n139 = Add Array Elements(numeric array=w307) -> (sum=w310:u32)
              n140 = Increment(x=w313) -> (x+1=w311:i32)
              n141 = Format Into String(format string="Ch.%2d: %d cnts.\t\t", initial string=w308, w311, w310) -> (resulting string=w309:string)  [unwired: 1 in, 1 out]
            }
            n142 = call "CalcRate.vi"("Refresh(ms)"=u32 100) -> ("Rate / Hz"=w279:dbl)  [unwired: 8 in, 2 out]
            n143 = Format Into String(format string="Readout Rate: %.1f Hz\\t\\t", w279) -> (resulting string=w288:string)  [unwired: 2 in, 1 out]
            n144 = for {
              tunnel: w280 -> [w305] mode=indexing
              tunnel: w279 -> [w304]
              tunnel: [w302] -> w278 mode=indexing
              tunnel: w271 -> [w303] mode=indexing
              tunnel: w269 -> [w301] mode=indexing
              tunnel: [w296] -> w265 mode=indexing
              tunnel: [w295] -> w267 mode=indexing
              tunnel: w268 -> [w299] mode=indexing
              n145 = Array Max & Min(array=w305) -> (max value=w302:u32)  [unwired: 3 out]
              n146 = Subtract(x=w302, y=w303) -> (x-y=w306:u32)
              n147 = local read "syncrate"() -> (w298:i32)
              n148 = Multiply(x=w306, y=w304) -> (x*y=w297:dbl)
              n149 = Divide(x=w297, y=w298) -> (x/y=w300:dbl)
              n150 = Build Array (concatenate)(w301, w297) -> (w296:dbl[])
              n151 = Build Array (concatenate)(w299, w300) -> (w295:dbl[])
            }
            n152 = Concatenate Strings(w288, w284) -> (w270:string)
            n153 = Bundle(0.0, "Resolution"=w276, "Histograms"=w280) -> (→"HistoGraph":T8)  [unwired: 1 in]
            n154 = local write "Status"(w270) -> ()
            n155 = First Call?() -> (First Call?: T/F=w262:bool)
            n156 = Bundle By Name(cluster=w274, "max value"=w278, "CoincidenceArray"=w265, "HR Array"=w267, "Clear Graph"=w262) -> (w275:T1)
            n157 = Delete From Array(array=w267, index (col)=0 ("index (row)")) -> (array with subset deleted=w261:dbl[][])  [unwired: 2 in, 1 out]
            n158 = Delete From Array(array=w265, index (col)=0 ("index (row)")) -> (array with subset deleted=→"Coincidence Array":dbl[][])  [unwired: 2 in, 1 out]
            n159 = for {
              tunnel: w261 -> [w291] mode=indexing
              tunnel: [w290] -> w260 mode=indexing
              n160 = for {
                tunnel: w291 -> [w294] mode=indexing
                tunnel: [w292] -> w290 mode=indexing
                n161 = Multiply(x=w294, y=100.0) -> (x*y=w292:dbl)
              }
            }
            "Heralding Ratio" <- w260
          }
        }
      }
      event "Start": Value Change {
        w323 = T6 2 items=["HIST"=0, "T2"=2, "T3"=3] ("y")
        n162 = event-data() -> ()  [unwired: 1 in, 6 out]
        n163 = Unbundle By Name(w325) -> ("Mode"=w324:T6)
        n164 = Equal?(x=w324, y=w323) -> (x = y?=w321:bool)
        n165 = case shown="True" "Start" {
          selector: "Start" -> [w336 w341]
          tunnel: w325 -> [w334 w342]
          tunnel: [w335 w340] -> w326
          tunnel: w321 -> [_ w343]
          tunnel: w320 -> [w333 w339]
          tunnel: [w332 w338] -> w319
          frame False {
            n166 = property class="VI"() -> (error out=w331:errorcluster, "Panel"=w329:refnum<vi>)  [unwired: 2 in, 1 out]
            n167 = Bundle By Name(cluster=w334, "Scanning"=FALSE, "StartMeas"=w336) -> (w335:T1)
            n168 = call "EnableControls.vi"("error in (no error)"=w331, "Disabled"=T10."Enabled", "Panel in"=w329) -> ()  [unwired: 8 in, 1 out]
            n169 = local read "Multiharp Enqueuer"() -> (w327:refnum<class "Message Enqueuer.lvclass">)
            n170 = call "Send StopMeasurement.vi"("error in (no error)"=w333, "Message Enqueuer"=w327) -> ("error out"=w332:errorcluster)  [unwired: 8 in, 1 out]
            n171 = local write "Start"(FALSE ("StartMeas")) -> ()
          }
          frame True {
            n172 = case shown="True" w343 {
              tunnel: w342 -> [w345 w380]
              tunnel: w341 -> [_ _]
              tunnel: [w344 w382] -> w340
              tunnel: w339 -> [w347 w381]
              tunnel: [w346 w364] -> w338
              frame False {
                n173 = Two Button Dialog(message="Multiharp should be set to T2 Mode for this Measurement", 2:"Set to T2" ("T button name (\"OK\")")) -> (T button?=w348:bool)  [unwired: 1 in]
                n174 = case shown="True" w348 {
                  tunnel: w347 -> [w353 w363]
                  tunnel: [w353 w355] -> w346
                  tunnel: w345 -> [w351 w361]
                  tunnel: [w351 w360] -> w344
                  frame False {
                    n175 = local write "Start"(FALSE ("StartMeas")) -> ()
                  }
                  frame True {
                    w362 = T6 2 items=["HIST"=0, "T2"=2, "T3"=3] ("Mode")
                    n176 = local read "Multiharp Enqueuer"() -> (w354:refnum<class "Message Enqueuer.lvclass">)
                    n177 = Bundle By Name(cluster=w361, "Mode"=w362) -> (w360:T1)
                    n178 = call "Send MH_Init.vi"("error in (no error)"=w363, "Mode"=w362, "Message Enqueuer"=w354) -> ("error out"=w356:errorcluster)  [unwired: 7 in, 1 out]
                    n179 = property class="VI"(error in=w356) -> (error out=w359:errorcluster, "Panel"=w357:refnum<vi>)  [unwired: 1 in, 1 out]
                    n180 = call "EnableControls.vi"("error in (no error)"=w359, "Disabled"=T10."Disabled and Grayed Out", "Panel in"=w357) -> ("error out"=w355:errorcluster)  [unwired: 8 in]
                  }
                }
              }
              frame True {
                w366 = T10."Enabled" ("Disabled")
                n181 = local read "FileName"() -> (w377:string)
                n182 = local read "Path"() -> (w376:path)
                n183 = local read "Acquisitions"() -> (w374:u32)
                n184 = Build Path(base path=w376, name or relative path=w377) -> (appended path=w379:path)
                n185 = Initialize Array(0 ("dimension size"), 1 ("dimension size"), 4 ("dimension size")) -> (w370:i32[][])
                n186 = local read "Multiharp Enqueuer"() -> (w368:refnum<class "Message Enqueuer.lvclass">)
                n187 = local read "VI"() -> (w367:refnum<vi>)
                n188 = Bundle By Name(cluster=w380, "Scanning"=TRUE, "File Save Path"=w379, "Acquisitions"=w374, "T2 Coincidences Array"=w370) -> (w378:T1)
                n189 = call "StartMeasurement.vi"("First Measurement?"=TRUE, "MH_UIThread_Data"=w378, "error in (no error)"=w381, "VI reference"=w367, "Multiharp Enqueuer"=w368) -> ("error out"=w365:errorcluster, "MH_UIThread_Data"=w382:T1)  [unwired: 5 in]
                n190 = property on="Start" class="Bool (strict)"(error in=w365, "DisabledEnum"=w366) -> (error out=w364:errorcluster)  [unwired: 1 in, 1 out]
                n191 = property on="T2 Coincidence Cluster.Coincidences" class="WFGraph (strict)"("DisabledEnum"=w366) -> ()  [unwired: 2 in, 2 out]
              }
            }
          }
        }
      }
      event User Event {
        w388 = T6 2 items=["HIST"=0, "T2"=2, "T3"=3] ("y")
        n192 = event-data() -> ("Last Move?"=w384:bool, "First Move?"=w383:bool)  [unwired: 1 in, 4 out]
        n193 = Unbundle By Name(w390) -> ("Mode"=w389:T6)
        n194 = Equal?(x=w389, y=w388) -> (x = y?=w387:bool)
        n195 = case shown="True" w387 {
          tunnel: w390 -> [w393 w419]
          tunnel: [w392 w414] -> w391
          tunnel: w386 -> [w395 w421]
          tunnel: [w394 w426] -> w385
          tunnel: w384 -> [_ _]
          tunnel: w383 -> [_ w420]
          frame False {
            # "Send Message that scan failed"
            n196 = Two Button Dialog(message="Multiharp should be set to T2 Mode for this Measurement", 2:"Set to T2" ("T button name (\"OK\")")) -> (T button?=w396:bool)  [unwired: 1 in]
            n197 = case shown="True" w396 {
              tunnel: w395 -> [w401 w407]
              tunnel: [w401 w403] -> w394
              tunnel: w393 -> [w400 w411]
              tunnel: [w400 w410] -> w392
              frame False {
                n198 = local write "Start"(FALSE ("StartMeas")) -> ()
              }
              frame True {
                w412 = T6 2 items=["HIST"=0, "T2"=2, "T3"=3] ("Mode")
                n199 = local read "Multiharp Enqueuer"() -> (w402:refnum<class "Message Enqueuer.lvclass">)
                n200 = Bundle By Name(cluster=w411, "Mode"=w412) -> (w410:T1)
                n201 = property class="VI"(error in=w407) -> (error out=w406:errorcluster, "Panel"=w409:refnum<vi>)  [unwired: 1 in, 1 out]
                n202 = call "Send MH_Init.vi"("error in (no error)"=w407, "Mode"=w412, "Message Enqueuer"=w402) -> ("error out"=w404:errorcluster)  [unwired: 7 in, 1 out]
                n203 = call "EnableControls.vi"("error in (no error)"=w406, "Disabled"=T10."Disabled and Grayed Out", "Panel in"=w409) -> ("error out"=w405:errorcluster)  [unwired: 8 in]
                n204 = Merge Errors(w405, w404) -> (w403:errorcluster)
              }
            }
          }
          frame True {
            w416 = T10."Enabled" ("Disabled")
            w427 = TRUE ("StartMeas")
            n205 = local read "FileName"() -> (w423:string)
            n206 = local read "Path"() -> (w424:path)
            n207 = Build Path(base path=w424, name or relative path=w423) -> (appended path=w425:path)
            n208 = local read "Multiharp Enqueuer"() -> (w413:refnum<class "Message Enqueuer.lvclass">)
            n209 = Bundle By Name(cluster=w419, "StartMeas"=w427, "Ext. Scanning"=w427, "File Save Path"=w425) -> (w418:T1)
            n210 = local read "VI"() -> (w417:refnum<vi>)
            n211 = call "StartMeasurement.vi"("First Measurement?"=w420, "MH_UIThread_Data"=w418, "error in (no error)"=w421, "VI reference"=w417, "Multiharp Enqueuer"=w413) -> ("error out"=w422:errorcluster, "MH_UIThread_Data"=w414:T1)  [unwired: 5 in]
            n212 = property on="stop" class="Bool"(error in=w422, "DisabledEnum"=w416) -> (error out=w415:errorcluster)  [unwired: 1 in, 1 out]
            n213 = property on="Init Multiharp" class="Bool"(error in=w415, "DisabledEnum"=w416) -> (error out=w426:errorcluster)  [unwired: 1 in, 1 out]
          }
        }
      }
      event User Event {
        w444 = FALSE ("Scanning")
        n214 = event-data() -> ()  [unwired: 1 in, 5 out]
        n215 = Bundle By Name(cluster=w446, "Scanning"=w444, "Ext. Scanning"=w444) -> (w443:T1)
        n216 = property class="VI"(error in=w445) -> (error out=w448:errorcluster, "Panel"=w449:refnum<vi>)  [unwired: 1 in, 1 out]
        n217 = Unbundle By Name(w443) -> ("File Save Path"=w441:path, "AllanVariance"=w432:dbl[][])
        n218 = call "EnableControls.vi"("error in (no error)"=w448, "Disabled"=T10."Enabled", "Panel in"=w449) -> ("error out"=w434:errorcluster)  [unwired: 8 in]
        n219 = Path To String(path=w441) -> (string=w440:string)
        n220 = Array To Spreadsheet String(delimiter (Tab)=",", array=w432, 3:"%.2f " ("format string")) -> (spreadsheet string=w431:string)
        n221 = Concatenate Strings(w440, "Allan.csv" ("string")) -> (w439:string)
        n222 = String To Path(string=w439) -> (path=w438:path)
        n223 = Open/Create/Replace File(file path (use dialog)=w438, error in=w434) -> (refnum out=w430:refnum<file>, error out=w435:errorcluster)  [unwired: 4 in, 1 out]
        n224 = Write to Text File(file (use dialog)=w430, text=w431, error in=w435) -> (refnum out=w437:refnum<file>, error out=w436:errorcluster)  [unwired: 1 in, 1 out]
        n225 = Close File(refnum=w437, error in=w436) -> (error out=w433:errorcluster)  [unwired: 1 out]
      }
      event "Channels": Value Change {
        n226 = event-data() -> ()  [unwired: 1 in, 1 out]
        n227 = Array Size(array="Channels") -> (size(s)=w462:i32)
        n228 = Unbundle By Name(w451) -> ("Channels"=w460:T3[], "Init Info.nchannels"=w463:i32, "DevIdx"=w452:i32, "Init Info.features"=w453:i32)
        n229 = Not Equal?(x=w463, y=w462) -> (x != y?=w461:bool)
        n230 = local read "AllChannels"() -> (w455:T9)
        n231 = case shown="False" w461 {
          tunnel: "Channels" -> [w470 _]
          tunnel: [w466 w504] -> w459
          tunnel: w460 -> [w471 w504]
          tunnel: [w465 _] -> w457
          tunnel: w455 -> [w469 w503]
          tunnel: [w468 w503] -> w454
          tunnel: w453 -> [w467 _]
          tunnel: w452 -> [_ _]
          frame False {
            n232 = call "MH_SetInputChannels.vi"("Channels new"=w470, "Channels old"=w471) -> ("SetInpChan"=w465:T4[], "Channels"=w466:T11[])  [unwired: 8 in]
            n233 = for {
              tunnel: w465 -> [w496] mode=indexing
              shift-right: [w478] -> w468
              shift-left: w469 -> [w480]
              n234 = Unbundle By Name(w480) -> ("SetEnableAllChan"=w489:bool, "SetEdgeAllChan"=w488:bool, "SetLevelAllChan"=w487:bool, "SetOffsetAllChan"=w486:bool, "SetUseDTAllChan"=w485:bool, "SetDeadTAllChan"=w484:bool)
              n235 = Unbundle By Name(w496) -> ("Changed.Enable"=w495:bool, "Changed.Edge"=w494:bool, "Changed.Level"=w493:bool, "Changed.Offset"=w492:bool, "Changed.UseDeadTime"=w491:bool, "Changed.DeadTime"=w490:bool)
              n236 = Build Array(w495, w494, w493, w492, w491, w490) -> (w482:bool[])
              n237 = Build Array(w489, w488, w487, w486, w485, w484) -> (w483:bool[])
              n238 = for {
                tunnel: w483 -> [w499] mode=indexing
                tunnel: w482 -> [w497] mode=indexing
                tunnel: [w498] -> w481 mode=indexing
                n239 = case shown="True" w499 {
                  selector: w499 -> [w500 _]
                  tunnel: [w500 w501] -> w498
                  tunnel: w497 -> [_ w502]
                  frame False {
                  }
                  frame True {
                    n240 = Not(x=w502) -> (.not. x?=w501:bool)
                  }
                }
              }
              n241 = Array To Cluster(array=w481) -> (cluster=w479:T13)
              n242 = Unbundle(w479) -> ("[0]"=w477:bool, "[1]"=w476:bool, "[2]"=w475:bool, "[3]"=w474:bool, "[4]"=w473:bool, "[5]"=w472:bool)
              n243 = Bundle By Name(cluster=w480, "SetEnableAllChan"=w477, "SetEdgeAllChan"=w476, "SetLevelAllChan"=w475, "SetOffsetAllChan"=w474, "SetUseDTAllChan"=w473, "SetDeadTAllChan"=w472) -> (w478:T9)
            }
            n244 = local read "Multiharp Enqueuer"() -> (w464:refnum<class "Message Enqueuer.lvclass">)
            n245 = call "Send SetInputChannels.vi"("Channels"=w466, "SetInpChan"=w465, "features"=w467, "Message Enqueuer"=w464) -> ()  [unwired: 6 in, 2 out]
          }
          frame True {
          }
        }
        n246 = local write "AllChannels"(w454) -> ()
        n247 = local write "Channels"(w459) -> ()
        n248 = Bundle By Name(cluster=w451, "Channels"=w459, "SetInpChan"=w457) -> (w458:T1)
      }
      event "SyncDivider": Value Change {
        n249 = event-data() -> ()  [unwired: 1 in, 1 out]
        n250 = Bundle By Name(cluster=w509, "SyncDivider"="SyncDivider") -> (w512:T1)
        n251 = Power Of 2(x="SyncDivider") -> (2^x=w511:dbl)
        n252 = To Long Integer(number=w511) -> (32bit integer=w507:i32)
        n253 = local read "Multiharp Enqueuer"() -> (w505:refnum<class "Message Enqueuer.lvclass">)
        n254 = call "Send SetSyncDivider.vi"("SyncDivider"=w507, "Message Enqueuer"=w505) -> ("error out"=w506:errorcluster)  [unwired: 8 in, 1 out]
        n255 = flat-sequence {
          tunnel: w506 -> [w513]
          tunnel: [w513] -> w508
          frame #0 {
            n256 = Wait (ms)(milliseconds to wait=u32 100) -> ()  [unwired: 1 out]
          }
        }
      }
      event "SyncOffset": Value Change {
        n257 = event-data() -> ()  [unwired: 1 in, 6 out]
        n258 = local read "Multiharp Enqueuer"() -> (w515:refnum<class "Message Enqueuer.lvclass">)
        n259 = case shown="Default" "SyncOffset" {
          selector: "SyncOffset" -> [w521 _ _]
          tunnel: [w521 99999 ("SyncOffset") -99999 ("SyncOffset")] -> w519
          frame Default {
          }
          frame 100000.. {
          }
          frame ..-100000 {
          }
        }
        n260 = call "Send SetSyncOffset.vi"("error in (no error)"=w517, "Offset"="SyncOffset", "Message Enqueuer"=w515) -> ()  [unwired: 7 in, 2 out]
        n261 = local write "SyncOffset"(w519) -> ()
        n262 = Bundle By Name(cluster=w516, "SyncOffset"=w519) -> (w520:T1)
      }
      event "SyncLevel", "SyncEdge": Value Change {
        # "Send SyncTrigger Message"
        n263 = event-data() -> ()  [unwired: 1 in, 6 out]
        n264 = local read "Multiharp Enqueuer"() -> (w525:refnum<class "Message Enqueuer.lvclass">)
        n265 = call "Send SetSyncTrigger.vi"("SyncLevel"="SyncLevel", "SyncEdge"="SyncEdge", "Message Enqueuer"=w525) -> ()  [unwired: 7 in, 2 out]
        n266 = Bundle By Name(cluster=w526, "SyncEdge"="SyncEdge", "SyncLevel"="SyncLevel") -> (w529:T1)
      }
      event "UseDeadTime", "SyncDeadTime": Value Change {
        w537 = 32  # FEATURE_PROG_TD
        n267 = event-data() -> ()  [unwired: 1 in, 6 out]
        n268 = Unbundle By Name(w534) -> ("DevIdx"=w541:i32, "Init Info.features"=w536:i32)
        n269 = Bundle By Name(cluster=w534, "UseDeadTime"="UseDeadTime", "SyncDeadTime"="SyncDeadTime") -> (w542:T1)
        n270 = And(x=w536, y=w537) -> (x .and. y?=w538:i32)
        n271 = Boolean To (0,1)(Boolean="UseDeadTime") -> (0, 1=w540:i16)
        n272 = To Long Integer(number=w540) -> (32bit integer=w539:i32)
        n273 = Not Equal To 0?(x=w538) -> (x != 0?=w535:bool)
        n274 = case shown="True" w535 {
          tunnel: [_ w545] -> w530
          tunnel: w541 -> [_ _]
          tunnel: "SyncDeadTime" -> [_ w546]
          tunnel: w539 -> [_ w547]
          tunnel: w531 -> [_ w544]
          frame False {
          }
          frame True {
            n275 = local read "Multiharp Enqueuer"() -> (w543:refnum<class "Message Enqueuer.lvclass">)
            n276 = call "Send SetSyncDeadTime.vi"("error in (no error)"=w544, "deadtime"=w546, "on"=w547, "Message Enqueuer"=w543) -> ("error out"=w545:errorcluster)  [unwired: 6 in, 1 out]
          }
        }
      }
      event "HistoOffset", "HistoLength", "Binning": Value Change {
        n277 = event-data() -> ("CtlRef"=w557:refnum<vi>, "NewVal"=w558:i32)  [unwired: 1 in, 4 out]
        n278 = property class="Num"(reference=w557) -> ("Label.Text"=w556:string)  [unwired: 1 in, 2 out]
        n279 = Scale By Power Of 2(n="Binning", x=10) -> (x*2^n=w550:i32)
        n280 = Divide(x=w550, y=1000) -> (x/y=w548:dbl)
        n281 = Bundle By Name(cluster=w553, "HistoOffset"="HistoOffset", "HistoLength"="HistoLength", "Binning"="Binning", "Resolution"=w548) -> (w561:T1)
        n282 = case shown="\"HistoLength\", Default" w556 {
          tunnel: w558 -> [w566 w571 w576]
          tunnel: w555 -> [w562 w568 w573]
          tunnel: [w563 w567 w572] -> w554
          frame "Binning" {
            n283 = local read "Multiharp Enqueuer"() -> (w564:refnum<class "Message Enqueuer.lvclass">)
            n284 = call "Send SetHistogramParameter.vi"("error in (no error)"=w562, "Value"=w566, "Parameter"=enum16{"HistoLen", "HistoOffset", "Binning"}."Binning", "Message Enqueuer"=w564) -> ("error out"=w563:errorcluster)  [unwired: 6 in, 1 out]
          }
          frame "HistoLength", Default {
            n285 = local read "Multiharp Enqueuer"() -> (w569:refnum<class "Message Enqueuer.lvclass">)
            n286 = call "Send SetHistogramParameter.vi"("error in (no error)"=w568, "Value"=w571, "Parameter"=enum16{"HistoLen", "HistoOffset", "Binning"}."HistoLen", "Message Enqueuer"=w569) -> ("error out"=w567:errorcluster)  [unwired: 6 in, 1 out]
          }
          frame "HistoOffset" {
            n287 = local read "Multiharp Enqueuer"() -> (w574:refnum<class "Message Enqueuer.lvclass">)
            n288 = call "Send SetHistogramParameter.vi"("error in (no error)"=w573, "Value"=w576, "Parameter"=enum16{"HistoLen", "HistoOffset", "Binning"}."HistoOffset", "Message Enqueuer"=w574) -> ("error out"=w572:errorcluster)  [unwired: 6 in, 1 out]
          }
        }
      }
      event "Histograms On": Value Change {
        w586 = T6 0 items=["HIST"=0, "T2"=2, "T3"=3] ("y")
        n289 = event-data() -> ()  [unwired: 1 in, 6 out]
        n290 = Unbundle By Name(w587) -> ("AcqTime"=w579:i32, "Mode"=w581:T6)
        n291 = Bundle By Name(cluster=w587, "Histo On"="Histograms On", "max value"=u32[] [0, 0, 0, 0]) -> (w585:T1)
        n292 = Equal?(x=w581, y=w586) -> (x = y?=w582:bool)
        n293 = case shown="True" "Histograms On" {
          tunnel: "Histograms On" -> [w593 w596]
          tunnel: w585 -> [w591 w600]
          tunnel: w584 -> [w589 w599]
          tunnel: [w591 w598] -> w583
          tunnel: w582 -> [_ w597]
          tunnel: w579 -> [_ w595]
          tunnel: [w590 w594] -> w578
          frame False {
            n294 = local read "Multiharp Enqueuer"() -> (w588:refnum<class "Message Enqueuer.lvclass">)
            n295 = local write "Histograms On"(FALSE ("StartMeas")) -> ()
            n296 = call "Send MH_SetHistoOnOff.vi"("error in (no error)"=w589, "HistoOn/Off"=w593, "Message Enqueuer"=w588) -> ("error out"=w590:errorcluster)  [unwired: 7 in, 1 out]
          }
          frame True {
            n297 = case shown="True" w597 {
              tunnel: w600 -> [w605 w622]
              tunnel: w599 -> [w604 w619]
              tunnel: [w603 w622] -> w598
              tunnel: w596 -> [_ w621]
              tunnel: w595 -> [_ w620]
              tunnel: [w601 w618] -> w594
              frame False {
                n298 = local write "Histograms On"(FALSE ("Histograms On")) -> ()
                n299 = Two Button Dialog(message="Multiharp should be set to Histogramming Mode for this Measurement", 2:"Set to Histo Mode" ("T button name (\"OK\")")) -> (T button?=w606:bool)  [unwired: 1 in]
                n300 = case shown="True" w606 {
                  tunnel: w604 -> [w610 w616]
                  tunnel: [w610 w615] -> w601
                  tunnel: w605 -> [w609 w613]
                  tunnel: [w609 w612] -> w603
                  frame False {
                  }
                  frame True {
                    w614 = T6 0 items=["HIST"=0, "T2"=2, "T3"=3] ("Mode")
                    n301 = local read "Multiharp Enqueuer"() -> (w611:refnum<class "Message Enqueuer.lvclass">)
                    n302 = Bundle By Name(cluster=w613, "Mode"=w614) -> (w612:T1)
                    n303 = call "Send MH_Init.vi"("error in (no error)"=w616, "Mode"=w614, "Message Enqueuer"=w611) -> ("error out"=w615:errorcluster)  [unwired: 7 in, 1 out]
                  }
                }
              }
              frame True {
                n304 = local read "Multiharp Enqueuer"() -> (w617:refnum<class "Message Enqueuer.lvclass">)
                n305 = call "Send MH_SetHistoOnOff.vi"("error in (no error)"=w619, "tacq"=w620, "HistoOn/Off"=w621, "Message Enqueuer"=w617) -> ("error out"=w618:errorcluster)  [unwired: 6 in, 1 out]
              }
            }
          }
        }
      }
      event "AcqTime": Value Change {
        n306 = event-data() -> ()  [unwired: 1 in, 6 out]
        n307 = Bundle By Name(cluster=w626, "AcqTime"="AcqTime") -> (w625:T1)
      }
      event "OvlLevel", "StopOvl.": Value Change {
        n308 = event-data() -> ()  [unwired: 1 in, 1 out]
        n309 = Unbundle By Name(w628) -> ("DevIdx"=w631:i32)
        n310 = call "MH_SetStopOverflow.vi"("stopcount"="OvlLevel", "StopOnOverflow"="StopOvl.", "devidx"=w631) -> ()  [unwired: 7 in, 2 out]
        n311 = Bundle By Name(cluster=w628, "StopOvl."="StopOvl.", "OvlLevel"="OvlLevel") -> (w632:T1)
      }
      event "AllChannels": Value Change {
        n312 = event-data() -> ()  [unwired: 1 in, 1 out]
        n313 = local read "Channels"() -> (w638:T3[])
        n314 = call "MH_SetAllChannels.vi"("MH_UIThread_Data"=w636, "AllChannels"="AllChannels", "Channels in"=w638) -> ("MH_UIThread_Data"=w635:T1)  [unwired: 8 in]
        n315 = Unbundle By Name(w635) -> ("Channels"=w634:T3[])
        n316 = local write "Channels"(w634) -> ()
      }
      event "Coincidence Delays", "Max Triggers", "Coincidence Window": Value Change {
        n317 = event-data() -> ()  [unwired: 1 in, 6 out]
        n318 = Bundle By Name(cluster=w639, "Coincidence Window"="Coincidence Window", "Max Triggers"="Max Triggers", "Coincidence Delays"="Coincidence Delays") -> (w644:T1)
      }
      event "Run continuously": Value Change {
        n319 = event-data() -> ()  [unwired: 1 in, 1 out]
        n320 = Number To Boolean Array(number="Run continuously") -> (Boolean array=w648:bool[])
        n321 = Delete From Array(array=w648, index=0) -> (deleted portion=w646:bool)  [unwired: 1 in, 1 out]
        n322 = Bundle By Name(cluster=w651, "Run cont."=w646) -> (w650:T1)
      }
      event "Scale": Value Change {
        n323 = event-data() -> ()  [unwired: 1 in, 1 out]
      }
      event "stop": Value Change {
        n324 = event-data() -> ()  [unwired: 1 in, 6 out]
        n325 = Two Button Dialog(message="Really quit?", 2:"Quit" ("T button name (\"OK\")")) -> (T button?=w654:bool)  [unwired: 1 in]
        n326 = case shown="True" w654 {
          frame False {
          }
          frame True {
            n327 = local read "Multiharp Enqueuer"() -> (w660:refnum<class "Message Enqueuer.lvclass">)
            n328 = local read "Self Enqueuer"() -> (w659:refnum<class "Message Enqueuer.lvclass">)
            n329 = call <vilib>:"Send Normal Stop.vi"("Message Enqueuer"=w659) -> ()  [unwired: 10 in, 1 out]
            n330 = call <vilib>:"Send Normal Stop.vi"("Message Enqueuer"=w660) -> ()  [unwired: 10 in, 1 out]
          }
        }
      }
      event User Event {
        n331 = event-data() -> ()  [unwired: 1 in, 5 out]
      }
      event Timeout {
        n332 = event-data() -> ()  [unwired: 1 in, 1 out]
      }
      event Panel Resize {
        n333 = event-data() -> ()  [unwired: 1 in, 1 out]
      }
      event Panel Close? {
        n334 = event-data() -> ()  [unwired: 1 in, 1 out]
        n335 = Two Button Dialog(message="Really quit?", 2:"Quit" ("T button name (\"OK\")")) -> (T button?=w671:bool)  [unwired: 1 in]
        n336 = case shown="True" w671 {
          frame False {
          }
          frame True {
            n337 = local read "Multiharp Enqueuer"() -> (w675:refnum<class "Message Enqueuer.lvclass">)
            n338 = local read "Self Enqueuer"() -> (w674:refnum<class "Message Enqueuer.lvclass">)
            n339 = call <vilib>:"Send Normal Stop.vi"("Message Enqueuer"=w674) -> ()  [unwired: 10 in, 1 out]
            n340 = call <vilib>:"Send Normal Stop.vi"("Message Enqueuer"=w675) -> ()  [unwired: 10 in, 1 out]
          }
        }
        n341 = event-data("Discard?"=TRUE) -> ()  [unwired: 1 in, 1 out]
      }
    }
  }
  n342 = Unregister For Events(event registration refnum=w15) -> ()  [unwired: 1 in, 1 out]
